vi "Calibration Main.vi"(8 "error in (no error)":errorcluster, 11 "Pump Calibration Config in":T1={"Settings"={"Cycle Period"=500.0, "Ismatech"={"VISA resource name"="", "Simulated?"=TRUE, "Pump Number"=1.0, "Reverse?"=FALSE}, "Masterflex"={"VISA resource name"="", "Simulated?"=TRUE, "Pump Number"=1.0, "Reverse?"=FALSE}, "Bronkhorst M13 Flow Meter"={"VISA resource name"="", "Simulated?"=TRUE}, "PID 2 Parameters"={"Input Device"=enum."Default", "Output Device"=enum."Default"}, "Bronkhorst M14"={"VISA resource name"="", "Simulated?"=FALSE}, "Tacmina Settings"={"Analog DAQ Task"="", "Digital DAQ Task"=""}, "KNF SIMDOS Settings"={"VISA resource name"="", "Simulated?"=TRUE}, "VICI M50 Settings"={"VISA resource name"="", "Simulated?"=TRUE, "Pump Letter"="", "Reverse?"=FALSE}, "FLOM Settings"={"VISA resource name"="", "Simulated?"=TRUE, "Pump Number"=0.0}, "Calibration Limits"={"Minimum (ml/min)"=0.0, "Maximum (ml/min)"=0.0, "Steps"=0.0}, "SSI PR Settings"={"VISA resource name"="", "Simulated?"=FALSE}}, "Flowmeter Output"=0.0, "Density"=0.0, "FL Temp"=0.0, "Speed %"=0.0, "File Refnum"=refnum, "Pump On?"=enum."Not Initialized"} {"Settings"."Masterflex"."Pump Number" min=1.0 max=20.0 step=1.0; "Settings"."Ismatech"."Pump Number" min=1.0 max=20.0 step=1.0}) -> (0 "error out":errorcluster, 3 "Pump Calibration Config out":T1={"Settings"={"Cycle Period"=500.0, "Ismatech"={"VISA resource name"="", "Simulated?"=TRUE, "Pump Number"=1.0, "Reverse?"=FALSE}, "Masterflex"={"VISA resource name"="", "Simulated?"=TRUE, "Pump Number"=1.0, "Reverse?"=FALSE}, "Bronkhorst M13 Flow Meter"={"VISA resource name"="", "Simulated?"=TRUE}, "PID 2 Parameters"={"Input Device"=enum."Default", "Output Device"=enum."Default"}, "Bronkhorst M14"={"VISA resource name"="", "Simulated?"=FALSE}, "Tacmina Settings"={"Analog DAQ Task"="", "Digital DAQ Task"=""}, "KNF SIMDOS Settings"={"VISA resource name"="", "Simulated?"=TRUE}, "VICI M50 Settings"={"VISA resource name"="", "Simulated?"=TRUE, "Pump Letter"="", "Reverse?"=FALSE}, "FLOM Settings"={"VISA resource name"="", "Simulated?"=TRUE, "Pump Number"=0.0}, "Calibration Limits"={"Minimum (ml/min)"=0.0, "Maximum (ml/min)"=0.0, "Steps"=0.0}, "SSI PR Settings"={"VISA resource name"="", "Simulated?"=FALSE}}, "Flowmeter Output"=0.0, "Density"=0.0, "FL Temp"=0.0, "Speed %"=0.0, "File Refnum"=refnum, "Pump On?"=enum."Not Initialized"} {"Settings"."Masterflex"."Pump Number" min=1.0 max=20.0 step=1.0; "Settings"."Ismatech"."Pump Number" min=1.0 max=20.0 step=1.0})   [LabVIEW 2018, in "Calibration.lvlib"]
uses:
  Pfizer Timed Seq/Software/Calibration VIs/Calibration.lvlib
  Pump Calibration Config.ctl
  Pfizer Timed Seq/Software/Ismatec ISM 831C/Controls/Ismatech Settings Cluster.ctl
  Pfizer Timed Seq/Software/Masterflex 7550-30/Controls/Settings Cluster.ctl
  Pfizer Timed Seq/Software/Bronkhorst M13 Flow Meter/Settings Cluster.ctl
  Pfizer Timed Seq/Software/Measure Instrument/PID Input Enum.ctl
  Pfizer Timed Seq/Software/Measure Instrument/PID 2 Output Enum.ctl
  Pfizer Timed Seq/Software/Mettler Toledo/Controls/Settings Cluster.ctl
  Pfizer Timed Seq/Software/Tacmina QI/Tacmina QI DAQ Setting.ctl
  Pfizer Timed Seq/Software/KNF Pump/Settings Cluster plus SIMDOS.ctl
  Pfizer Timed Seq/Software/VICI M50 Party Mode/Settings Cluster.ctl
  Pfizer Timed Seq/Software/FLOM Pump/Settings Cluster.ctl
  Pfizer Timed Seq/Software/SSI PR Class/SSI PR Settings Cluster.ctl
  Pfizer Timed Seq/Software/Bronkhorst M14 Flow Meter/Settings Cluster.ctl
  Pfizer Timed Seq/Software/ASIA Pump/Pump Settings.ctl
  <vilib>/Platform/TimedLoop/XDataNode/timing_clust.ctl
  <vilib>/Platform/TimedLoop/XDataNode/nitl_modes.ctl
  <vilib>/Platform/TimedLoop/XDataNode/wakeup.ctl
  Pfizer Timed Seq/Software/support/Message Queue/Enqueue Message (Single).vi
  <vilib>/Utility/file.llb/Read Delimited Spreadsheet (string).vi
  <vilib>/Utility/file.llb/Write Delimited Spreadsheet (string).vi
  <vilib>/Platform/TimedLoop/XDataNode/XDataNode.xnode
  <vilib>/regexp/Match Regular Expression.xnode
  Pfizer Timed Seq/Software/KNF Pump/KNF SIMDOS.lvlib
  Pfizer Timed Seq/Software/Ismatec ISM 831C/Ismatec ISM 831C.lvlib
  Pfizer Timed Seq/Software/VICI M50 Party Mode/VICI M6 M50 Party Mode.lvlib
  Pfizer Timed Seq/Software/Masterflex 7550-30/Masterflex 7550-30.lvlib
  Pfizer Timed Seq/Software/FLOM Pump/FLOM Pump.lvlib
  Pfizer Timed Seq/Software/Bronkhorst M13 Flow Meter/Bronkhorst M13 Flow Meter.lvlib
  Pfizer Timed Seq/Software/Bronkhorst M14 Flow Meter/Bronkhorst M14 Flow Meter.lvlib
  Pfizer Timed Seq/Software/support/Message Queue/Message Queue.lvlib
  Pfizer Timed Seq/Software/SSI PR Class/SSI PR Pump.lvlib
  Support/Engine.lvlib
  <vilib>/Analysis/NI_AALPro.lvlib
  <vilib>/Platform/TimedLoop/XDataNode/XDNodeRunTimeDep.lvlib
  Pfizer Timed Seq/Software/Mettler Toledo/Mettler Toledo.lvlib
  Pfizer Timed Seq/Software/Tacmina QI/Tacmina QI.lvlib
  Pfizer Timed Seq/Software/ASIA Pump.lvlib
panel:
  out "Y array":dbl[](array[numeric])
  out "X array":dbl[](array[numeric])
  out "Output Selected":bool
  out "Input Selected":bool
  out "Step Array":dbl[](array[numeric])
  in  "?":enum32{"Settings", "Results"}(tab)
  in  "Settings Dialog":T15={"Cycle Period"=500.0, "Ismatech"={"VISA resource name"="", "Simulated?"=FALSE, "Pump Number"=1.0, "Reverse?"=FALSE}, "Masterflex"={"VISA resource name"="", "Simulated?"=FALSE, "Pump Number"=1.0, "Reverse?"=FALSE}, "Mettler"={"VISA resource name"="", "Simulated?"=FALSE}, "Bronkhorst M13 Flow Meter"={"VISA resource name"="", "Simulated?"=FALSE}, "Setup Parameters"={"Input Device"=enum."Default", "Output Device"=enum."Default"}, "Bronkhorst M14 Settings"={"VISA resource name"="", "Simulated?"=FALSE}, "Tacmina Settings"={"Analog DAQ Task"="", "Digital DAQ Task"=""}, "KNF SIMDOS Settings"={"VISA resource name"="", "Simulated?"=FALSE}, "ASIA Pump C"={"ASIA Pump #"=-1, "channel"=-1, "Simulated"=FALSE}, "VICI M50 Settings"={"VISA resource name"="", "Simulated?"=FALSE, "Pump Letter"="", "Reverse?"=FALSE}, "FLOM Settings"={"VISA resource name"="", "Simulated?"=FALSE, "Pump Number"=1.0}, "Calibration Limits"={"Minimum (ml/min)"=0.0, "Maximum (ml/min)"=0.0, "Steps"=0.0}, "File Name"="", "SSI PR Settings"={"VISA resource name"="", "Simulated?"=FALSE}} {"Calibration Limits"."Maximum (ml/min)" max=16.5; "ASIA Pump C"."channel" min=-1 max=1 step=1; "Masterflex"."Pump Number" min=1.0 max=20.0 step=1.0; "Ismatech"."Pump Number" min=1.0 max=20.0 step=1.0}
  in  "Start Button":bool
  in  "Cancel Button":bool
  out "Y Intercept":dbl
  in  "Accept Button":bool
  in  "Decline Button":bool
  out "Calibration Graph":cluster{dbl[], dbl[]}[](graph)
  out "Calibration Slope":dbl
  out "R^2 Value":dbl format="%#.4g"
  out "Pump Status":enum16{"Off", "On", "Not Initialized"}(ring)
  # "Output Instruments"
  # "Input Instruments"
  # "Output Instruments"
  # "Input Instruments"
  # "Output Instruments"
  # "Input Instruments"
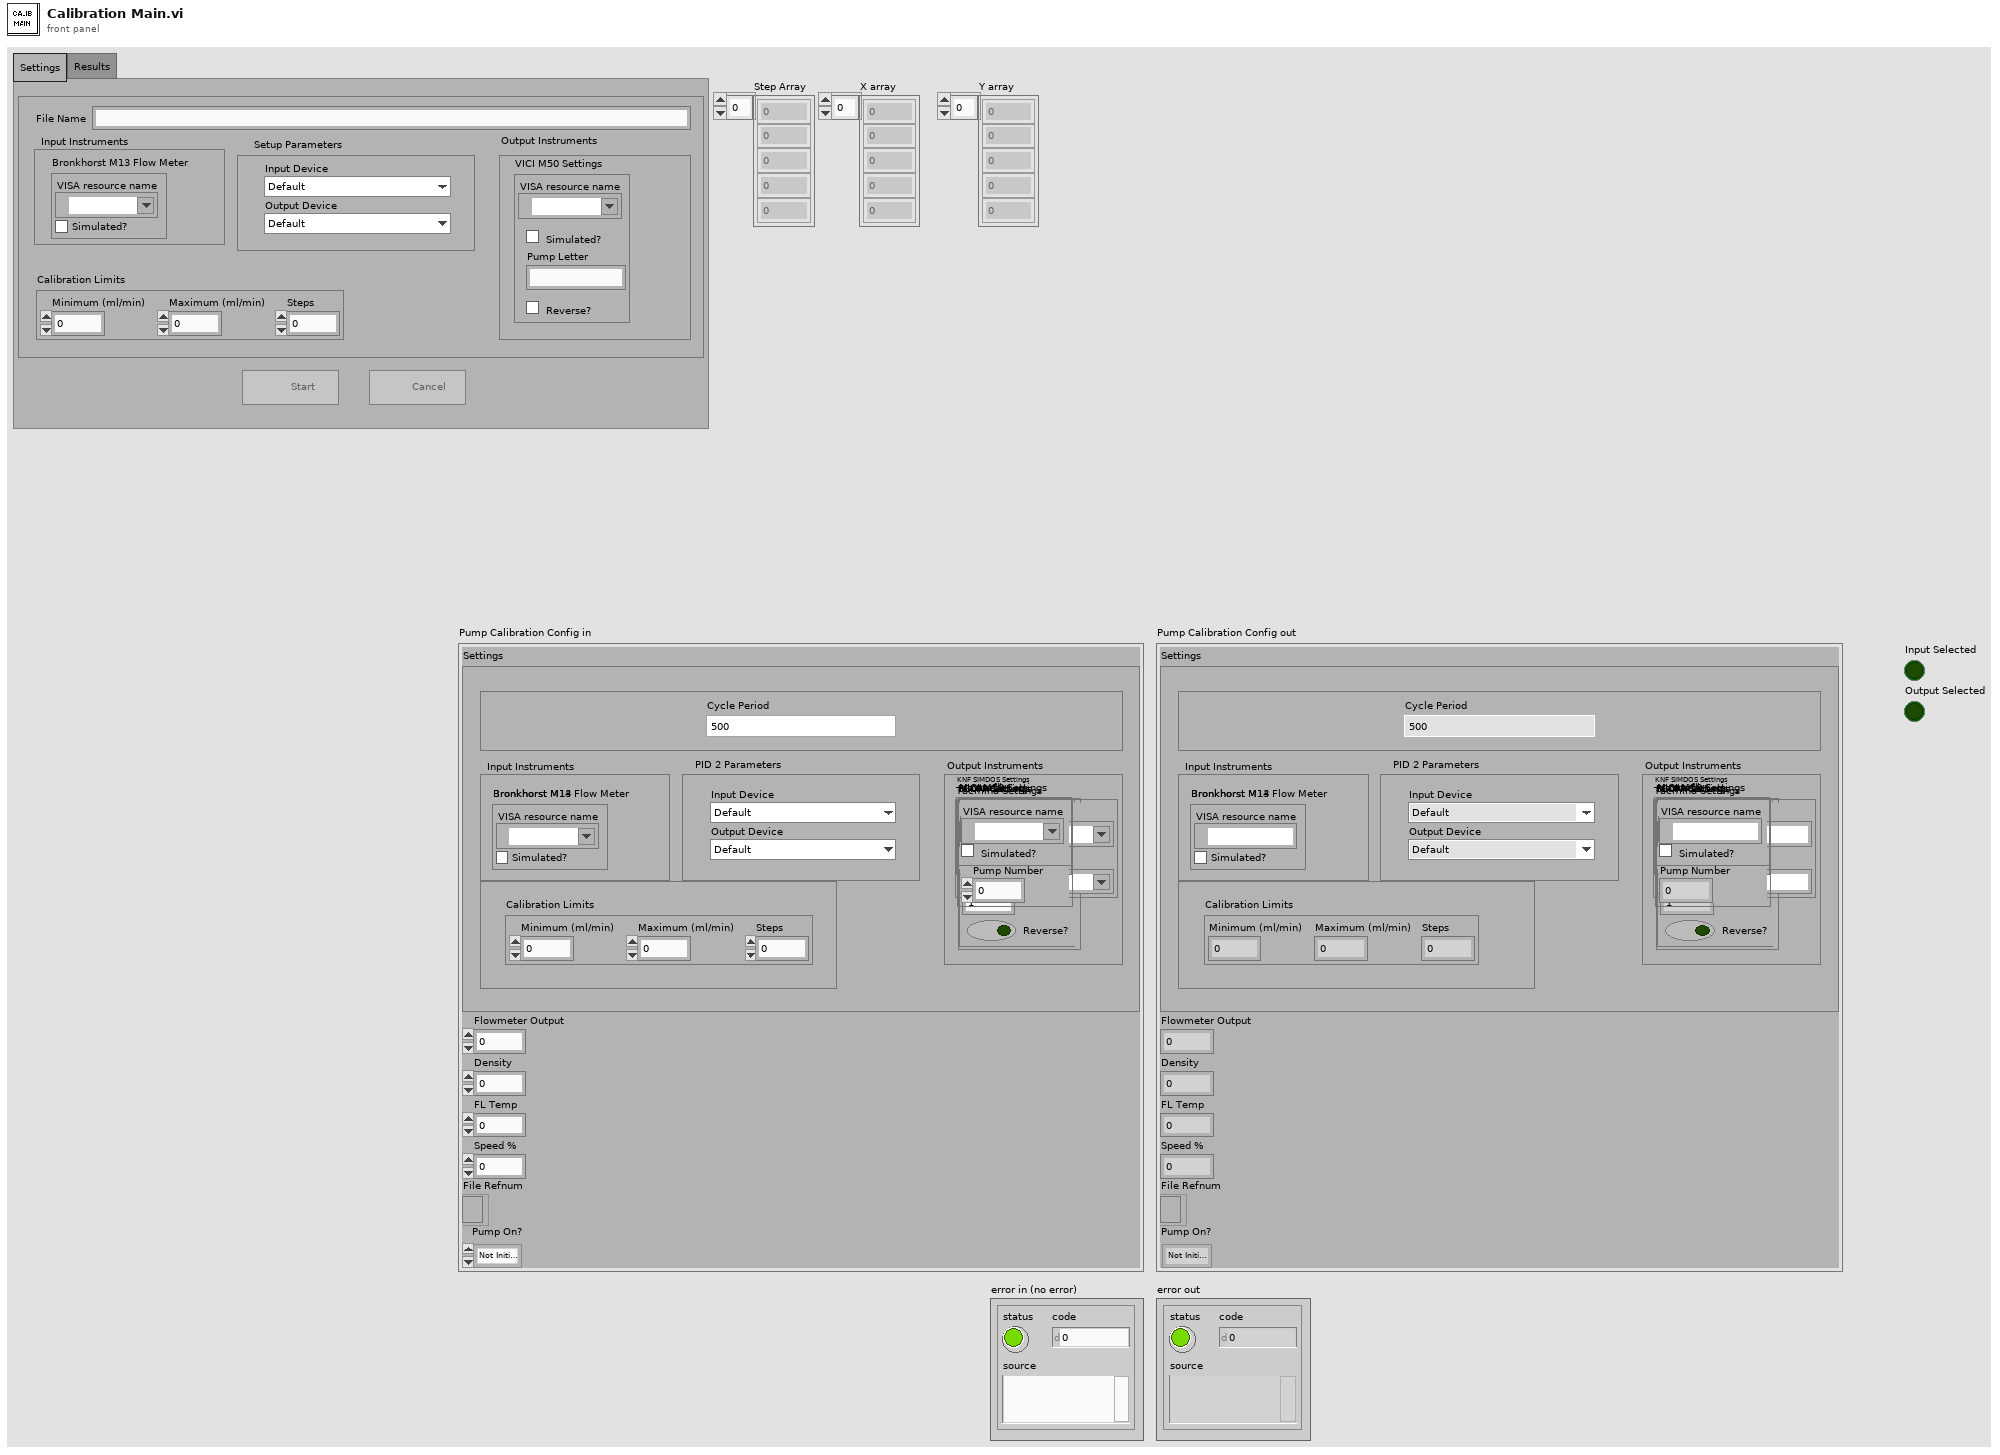
[diagram p1: front panel]
types:
  T1 = typedef "Calibration.lvlib/Pump Calibration Config.ctl" = cluster{"Settings":cluster{"Cycle Period":dbl, "Ismatech":T2, "Masterflex":T3, "Bronkhorst M13 Flow Meter":T4, "PID 2 Parameters":cluster{"Input Device":T5, "Output Device":T6}, "Bronkhorst M14":T7, "Tacmina Settings":T8, "KNF SIMDOS Settings":T9, "VICI M50 Settings":T10, "FLOM Settings":T11, "Calibration Limits":cluster{"Minimum (ml/min)":dbl, "Maximum (ml/min)":dbl, "Steps":dbl}, "SSI PR Settings":T12}, "Flowmeter Output":dbl, "Density":dbl, "FL Temp":dbl, "Speed %":dbl, "File Refnum":refnum<file>, "Pump On?":enum16{"Off", "On", "Not Initialized"}}
  T2 = typedef "Ismatec ISM 831C.lvlib/Ismatech Settings Cluster.ctl" = cluster{"VISA resource name":refnum<visa-resource-name>, "Simulated?":bool, "Pump Number":dbl, "Reverse?":bool}
  T3 = typedef "Masterflex 7550-30.lvlib/Settings Cluster.ctl" = cluster{"VISA resource name":refnum<visa-resource-name>, "Simulated?":bool, "Pump Number":dbl, "Reverse?":bool}
  T4 = typedef "Bronkhorst M13 Flow Meter.lvlib/Settings Cluster.ctl" = cluster{"VISA resource name":refnum<visa-resource-name>, "Simulated?":bool}
  T5 = typedef "PID Input Enum.ctl" = enum16{"Default", "Bronkhorst M13", "Bronkhorst M14", "Scale Rate of Change"}
  T6 = typedef "PID 2 Output Enum.ctl" = enum16{"Default", "Ismatec ISM 831C", "Masterflex 7550-30", "VICI", "Tacmina QI", "KNF SIMDOS", "ASIA Type C", "FLOM UI-22-11", "SSI PR"}
  T7 = typedef "Mettler Toledo.lvlib/Settings Cluster.ctl" = cluster{"VISA resource name":refnum<visa-resource-name>, "Simulated?":bool}
  T8 = typedef "Tacmina QI.lvlib/Tacmina QI DAQ Setting.ctl" = cluster{"Analog DAQ Task":refnum<k21>, "Digital DAQ Task":refnum<k21>}
  T9 = typedef "KNF SIMDOS.lvlib/Settings Cluster plus SIMDOS.ctl" = cluster{"VISA resource name":refnum<visa-resource-name>, "Simulated?":bool}
  T10 = typedef "VICI M6 M50 Party Mode.lvlib/Settings Cluster.ctl" = cluster{"VISA resource name":refnum<visa-resource-name>, "Simulated?":bool, "Pump Letter":string, "Reverse?":bool}
  T11 = typedef "FLOM Pump.lvlib/Settings Cluster.ctl" = cluster{"VISA resource name":refnum<visa-resource-name>, "Simulated?":bool, "Pump Number":dbl}
  T12 = typedef "SSI PR Pump.lvlib/SSI PR Settings Cluster.ctl" = cluster{"VISA resource name":refnum<visa-resource-name>, "Simulated?":bool}
  T13 = typedef "Bronkhorst M14 Flow Meter.lvlib/Settings Cluster.ctl" = cluster{"VISA resource name":refnum<visa-resource-name>, "Simulated?":bool}
  T14 = typedef "ASIA Pump.lvlib/Pump Settings.ctl" = cluster{"ASIA Pump #":i32, "channel":i32, "Simulated":bool}
  T15 = cluster{"Cycle Period":dbl, "Ismatech":T2, "Masterflex":T3, "Mettler":T7, "Bronkhorst M13 Flow Meter":T4, "Setup Parameters":cluster{"Input Device":T5, "Output Device":T6}, "Bronkhorst M14 Settings":T13, "Tacmina Settings":T8, "KNF SIMDOS Settings":T9, "ASIA Pump C":T14, "VICI M50 Settings":T10, "FLOM Settings":T11, "Calibration Limits":cluster{"Minimum (ml/min)":dbl, "Maximum (ml/min)":dbl, "Steps":dbl}, "File Name":string, "SSI PR Settings":T12}
  T16 = enum8{"Enabled", "Disabled", "Disabled and Grayed Out"}
  T17 = cluster{"Calibration UI":refnum<queue>, "Calibration Engine":refnum<queue>}
  T18 = typedef "XDNodeRunTimeDep.lvlib/timing_clust.ctl" = cluster{"Expected End [f-1]":u64, "Actual End [f-1]":u64, "Finished Late? [f-1]":bool, "Expected End [i-1]":u64, "Actual End [i-1]":u64, "Finished Late? [i-1]":bool, "Expected Start [i]":u64, "Actual Start [i]":u64, "Expected Start [f]":u64, "Actual Start [f]":u64, "Source Name":string, "Structure Name":string, "Period":i64, "Deadline":i64, "Offset":i64, "Start":i64, "Priority":i32, "Timeout":i32, "Mode":T19, "Wakeup Reason":T20, "Error":errorcluster, "Source Type":string, "Secondary Source Type":string, "Global End Time":u64, "Global Start Time":u64, "Frame Duration":u64, "Iteration Duration":u64, "Assigned CPU":i32, "I/O Scan Engine Mode":u32}
  T19 = typedef "XDNodeRunTimeDep.lvlib/nitl_modes.ctl" = enum32{"No Change", "Process missed periods, maintain original phase", "Discard missed periods, maintain original phase", "Process missed periods, ignore original phase", "Discard missed periods, ignore original phase"}
  T20 = typedef "XDNodeRunTimeDep.lvlib/wakeup.ctl" = enum32{"Normal", "Aborted", "Asynchronous wakeup", "Timing source error", "Timed loop error", "Timeout"}
  T21 = enum16{"open", "replace", "create", "open or create", "replace or create", "replace or create with confirmation"}
  T22 = cluster{"slope min":dbl, "slope max":dbl, "intercept min":dbl, "intercept max":dbl}
  T23 = cluster{"Minimum (ml/min)":dbl, "Maximum (ml/min)":dbl, "Steps":dbl}
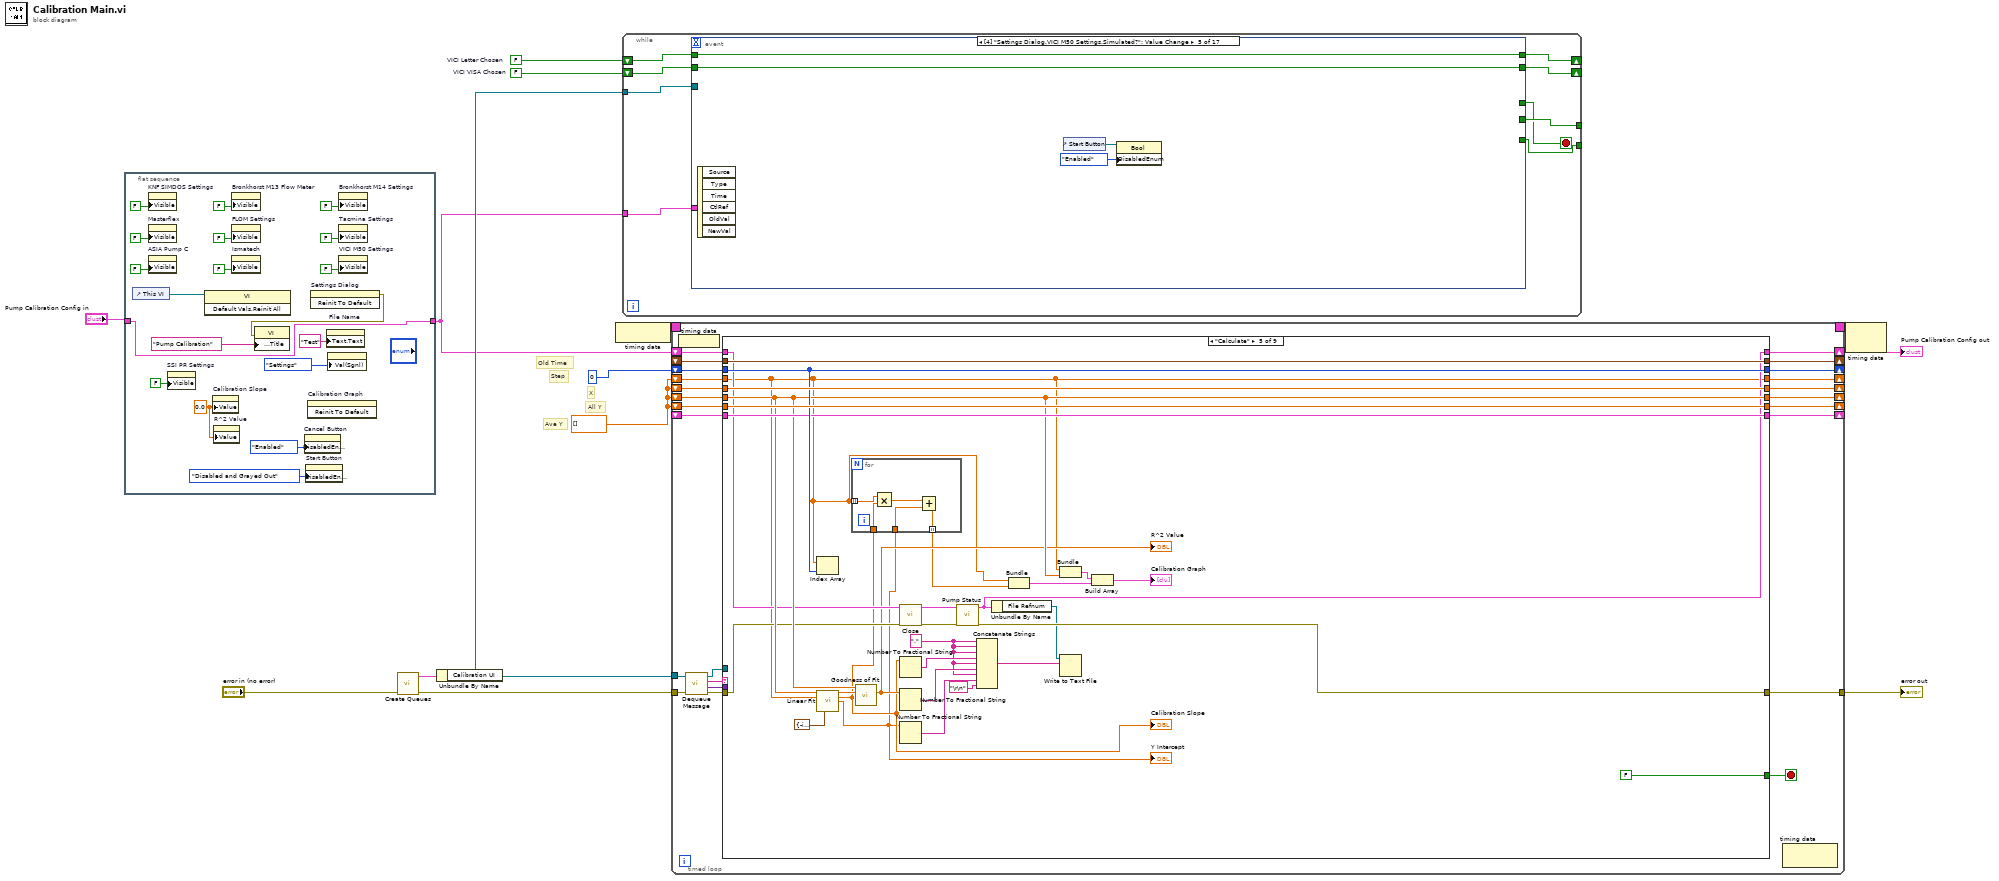
[diagram p0: block diagram]
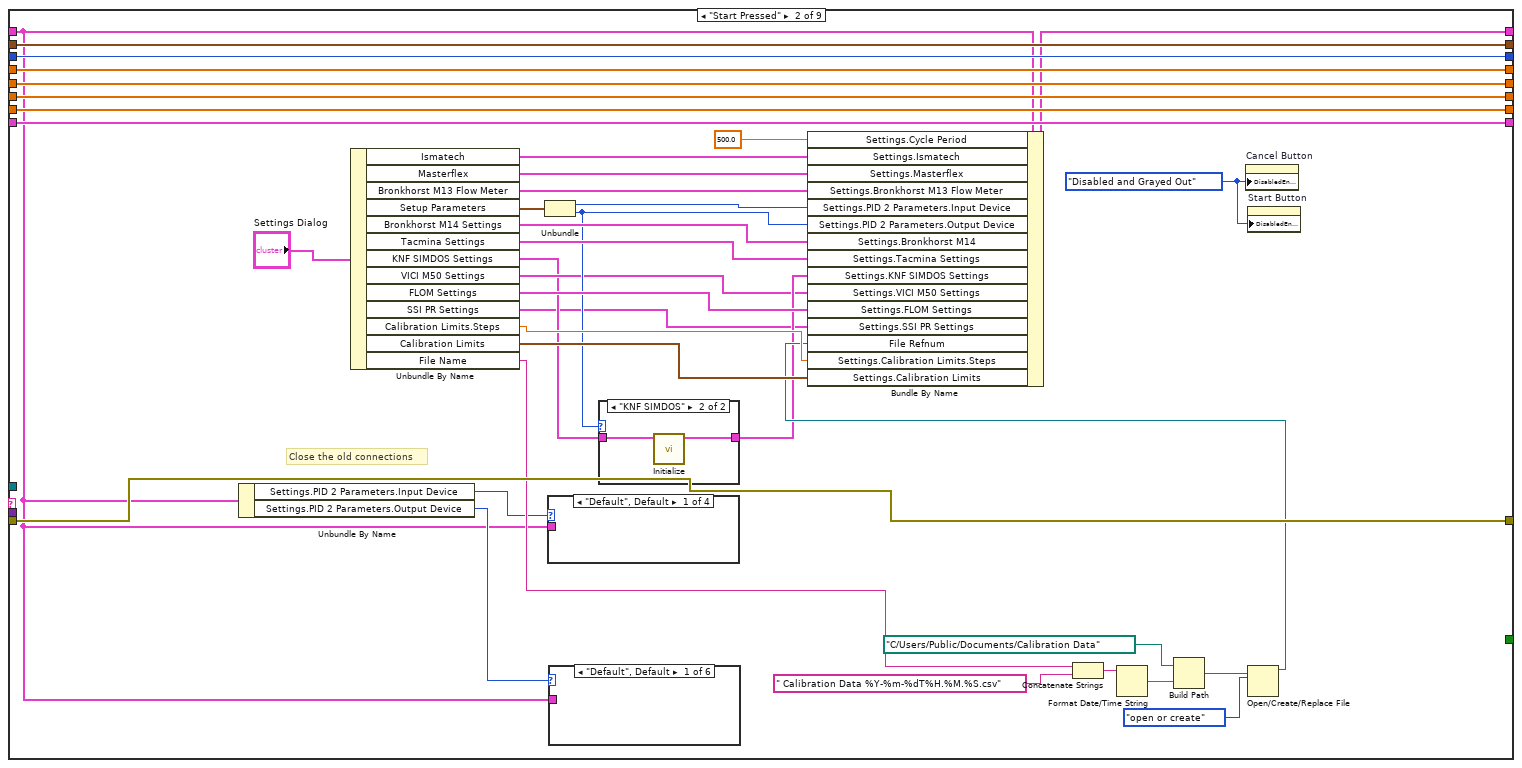
[diagram p3: hidden frame]
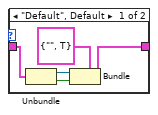
[diagram p4: hidden frame]
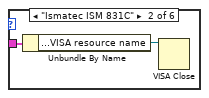
[diagram p5: hidden frame]
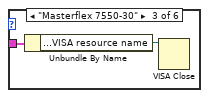
[diagram p6: hidden frame]
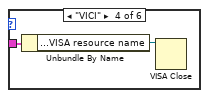
[diagram p7: hidden frame]
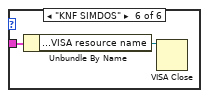
[diagram p9: hidden frame]
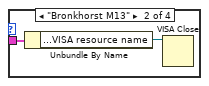
[diagram p10: hidden frame]
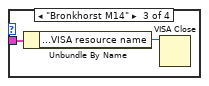
[diagram p11: hidden frame]
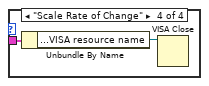
[diagram p12: hidden frame]
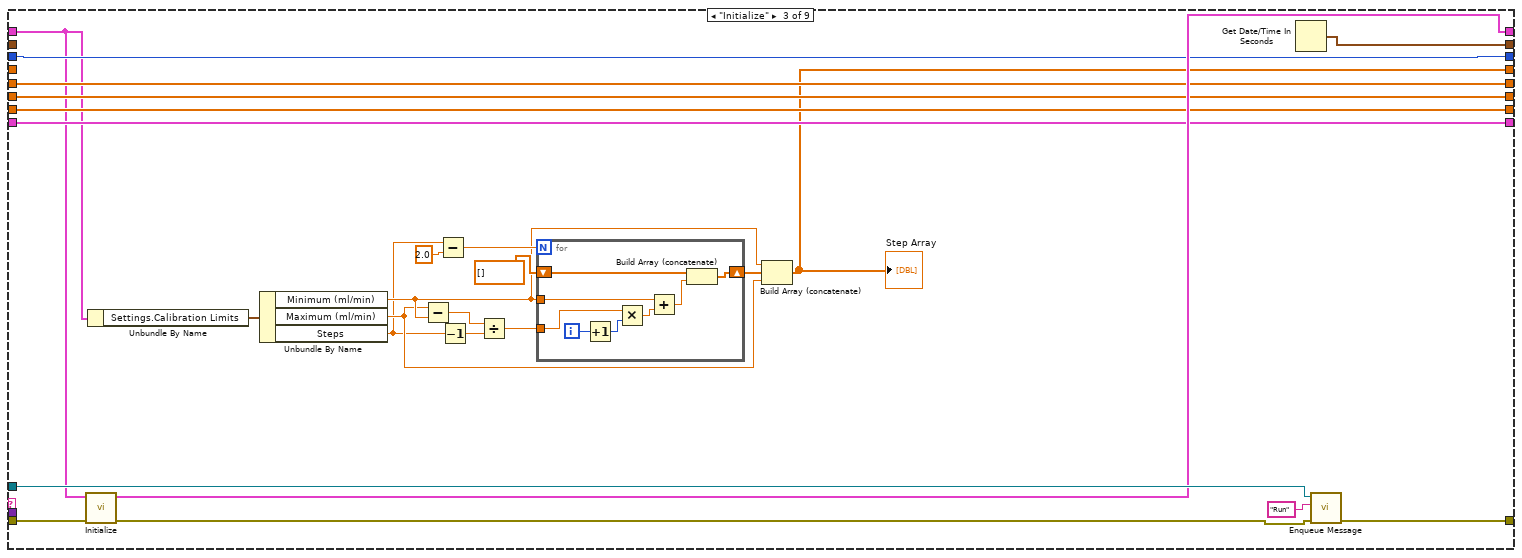
[diagram p13: hidden frame]
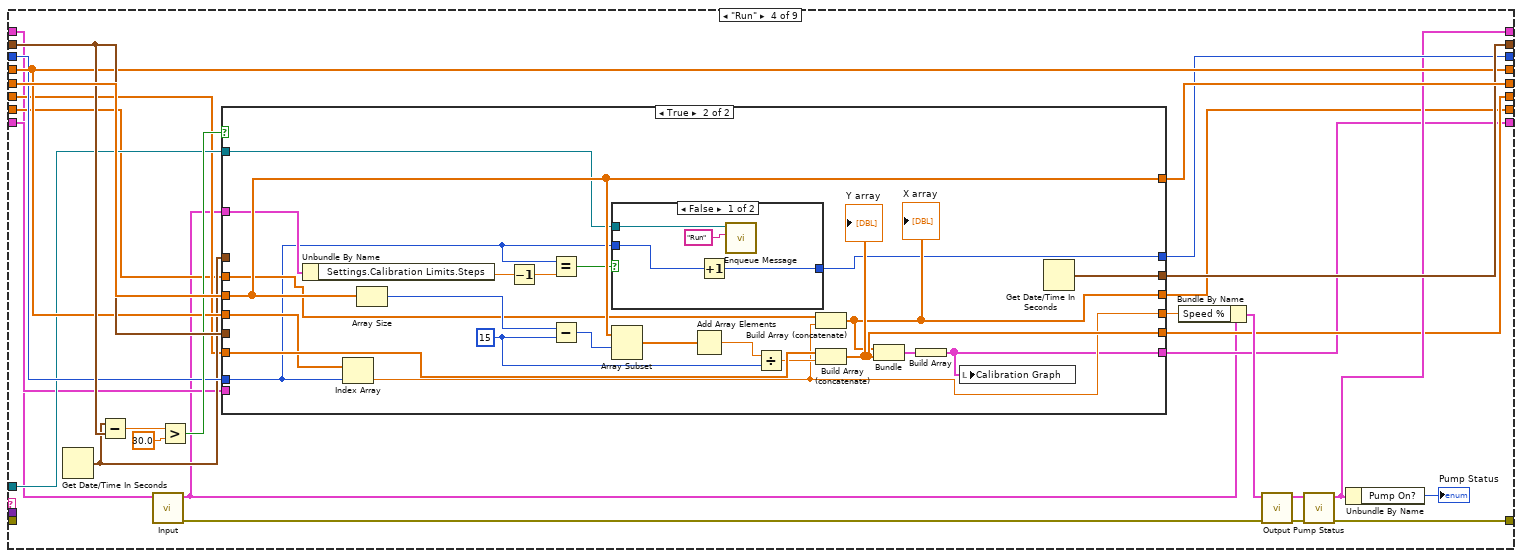
[diagram p14: hidden frame]
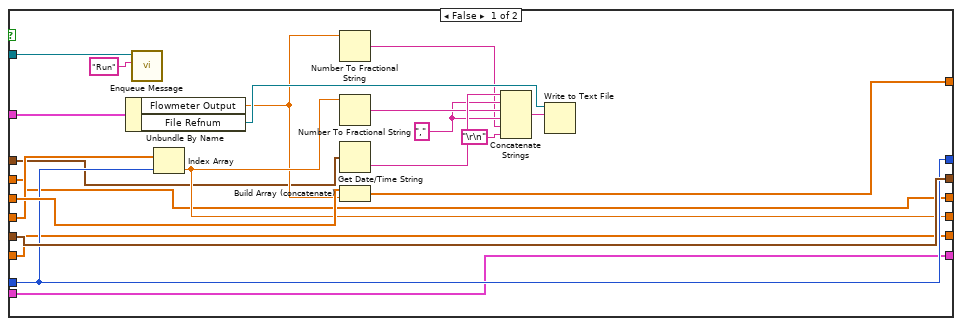
[diagram p15: hidden frame]
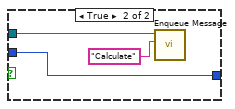
[diagram p16: hidden frame]
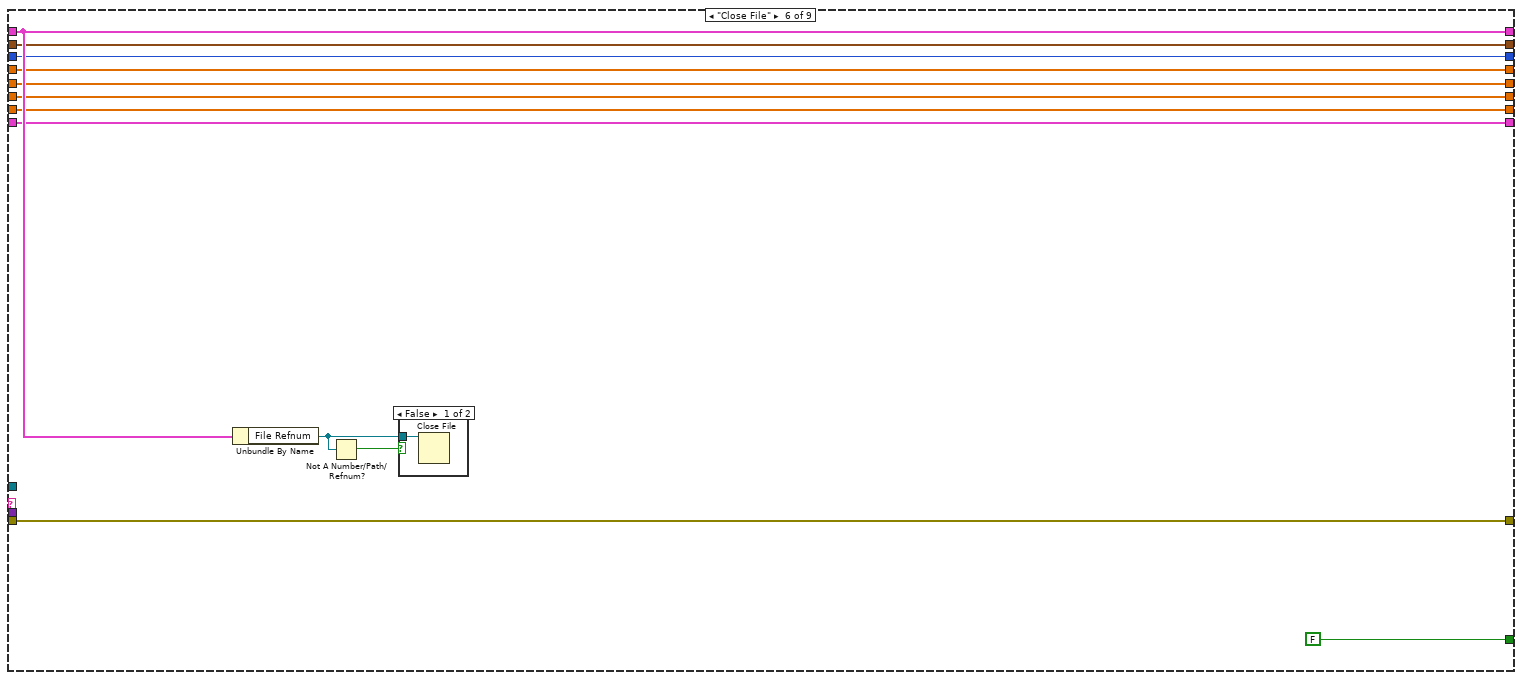
[diagram p17: hidden frame]
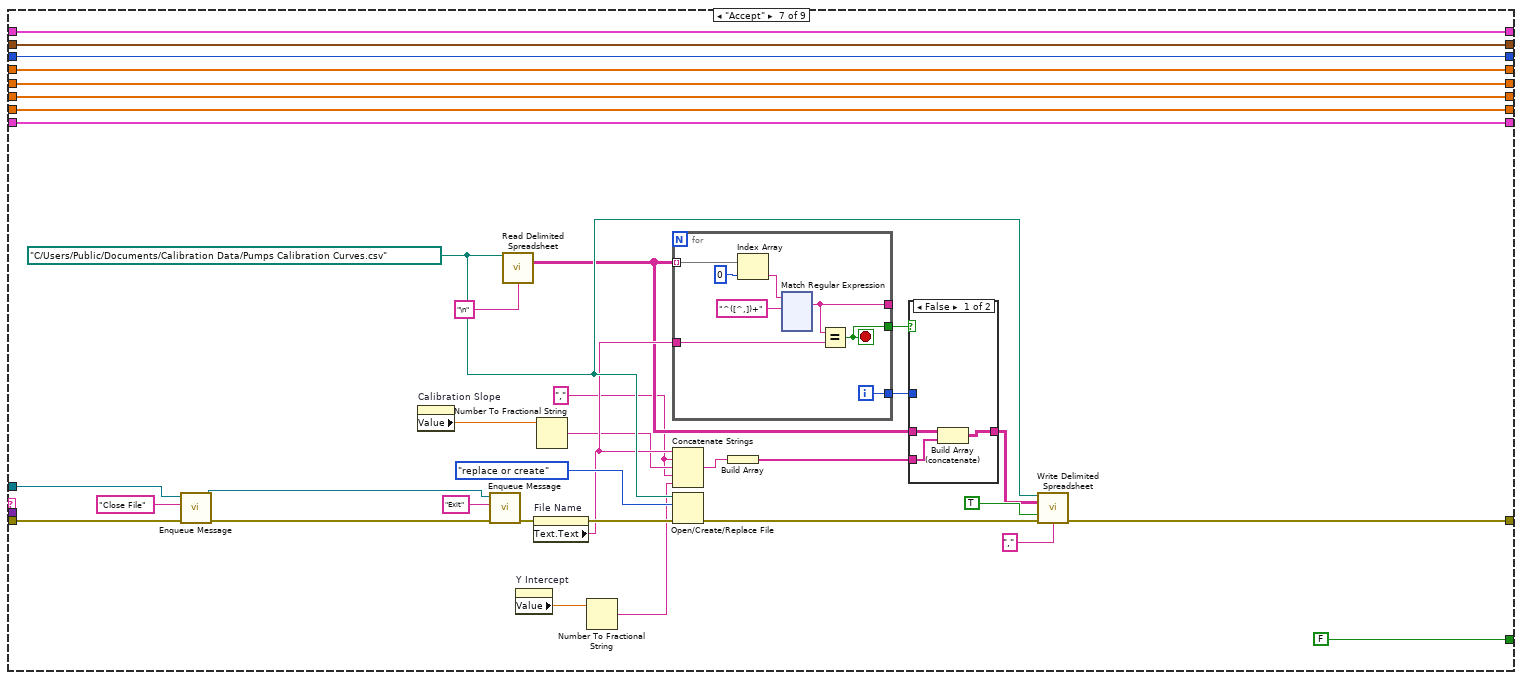
[diagram p19: hidden frame]
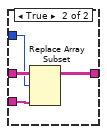
[diagram p20: hidden frame]
diagram:
  w1 = dbl[] []
  w13 = FALSE  # VICI VISA Chosen
  w14 = FALSE  # VICI Letter Chosen
  # "Old Time"
  # "Step"
  # "Ave Y"
  # "All Y"
  # "X"
  n1 = flat-sequence {
    tunnel: "Pump Calibration Config in" -> [w33]
    tunnel: [w33] -> w8
    frame #0 {
      w28 = 0.0 ("Calibration Slope")
      n2 = control-ref of="This VI"() -> (w27:refnum<vi>)
      n3 = property on="KNF SIMDOS Settings" class="Clust (strict)"("Visible"=FALSE) -> ()  [unwired: 2 in, 2 out]
      n4 = property on="Masterflex" class="Clust (strict)"("Visible"=FALSE) -> ()  [unwired: 2 in, 2 out]
      n5 = property on="ASIA Pump C" class="Clust (strict)"("Visible"=FALSE) -> ()  [unwired: 2 in, 2 out]
      n6 = property on="SSI PR Settings" class="Clust (strict)"("Visible"=FALSE) -> ()  [unwired: 2 in, 2 out]
      n7 = invoke class="VI" method="Default Vals.Reinit All"(reference=w27) -> ()  [unwired: 2 in, 3 out]
      n8 = property on="Calibration Slope" class="DigNum (strict)"("Value"=w28) -> ()  [unwired: 2 in, 2 out]
      n9 = property on="R^2 Value" class="DigNum (strict)"("Value"=w28) -> ()  [unwired: 2 in, 2 out]
      n10 = property on="Bronkhorst M13 Flow Meter" class="Clust (strict)"("Visible"=FALSE) -> ()  [unwired: 2 in, 2 out]
      n11 = property on="FLOM Settings" class="Clust (strict)"("Visible"=FALSE) -> ()  [unwired: 2 in, 2 out]
      n12 = property on="Ismatech" class="Clust (strict)"("Visible"=FALSE) -> ()  [unwired: 2 in, 2 out]
      n13 = property on="Cancel Button" class="Bool"("DisabledEnum"=T16."Enabled" ("Disabled")) -> ()  [unwired: 2 in, 2 out]
      n14 = property on="Start Button" class="Bool"("DisabledEnum"=T16."Disabled and Grayed Out" ("Disabled")) -> ()  [unwired: 2 in, 2 out]
      n15 = invoke on="Calibration Graph" class="XYGraph (strict)" method="Reinit To Default"() -> ()  [unwired: 3 in, 3 out]
      n16 = invoke on="Settings Dialog" class="Clust (strict)" method="Reinit To Default"() -> (error out=w30:errorcluster)  [unwired: 3 in, 2 out]
      n17 = property class="VI"(error in=w30, "Front Panel.Title"="Pump Calibration" ("string")) -> ()  [unwired: 1 in, 2 out]
      n18 = property on="File Name" class="Str"("Text.Text"="Test") -> ()  [unwired: 2 in, 2 out]
      n19 = property class="TabCtl (strict)"("Val(Sgnl)"=enum32{"Settings", "Results"}."Settings") -> ()  [unwired: 2 in, 2 out]
      n20 = property on="Bronkhorst M14 Settings" class="Clust (strict)"("Visible"=FALSE) -> ()  [unwired: 2 in, 2 out]
      n21 = property on="Tacmina Settings" class="Clust (strict)"("Visible"=FALSE) -> ()  [unwired: 2 in, 2 out]
      n22 = property on="VICI M50 Settings" class="Clust (strict)"("Visible"=FALSE) -> ()  [unwired: 2 in, 2 out]
    }
  }
  n23 = call "Create Queues.vi"("error in (no error)"="error in (no error)") -> ("error out"=w6:errorcluster, "Message Queues Out"=w10:T17)  [unwired: 9 in]
  n24 = Unbundle By Name(w10) -> ("Calibration UI"=w9:refnum<queue>)
  n25 = node-c288() -> (w4:T18)
  n26 = while {
    tunnel: [w42] -> _
    tunnel: [w40] -> _
    shift-right: [w39] -> _
    shift-left: w14 -> [w38]
    shift-right: [w37] -> _
    shift-left: w13 -> [w36]
    tunnel: w8 -> [w34]
    tunnel: w9 -> [w35]
    stop <- w41 stop-if-true
    n27 = event shown="[4] \"Settings Dialog.VICI M50 Settings.Simulated?\": Value Change" {
      selector: _ -> [_ _ _ _ _ _ _ _ _ _ _ _ _ _ _ _ _]
      dyn-events: _ -> [_ _ _ _ _ _ _ _ _ _ _ _ _ _ _ _ _]
      timeout: _ -> [_ _ _ _ _ _ _ _ _ _ _ _ _ _ _ _ _]
      tunnel: [FALSE ("UI Refresh Needed?") _ _ _ _ _ _ _ _ _ _ _ _ _ FALSE ("UI Refresh Needed?") FALSE ("UI Refresh Needed?") FALSE ("UI Refresh Needed?")] -> w42
      tunnel: [FALSE _ _ _ _ _ _ _ _ _ _ _ _ _ TRUE TRUE TRUE] -> w41
      tunnel: [FALSE ("UI Refresh Needed?") _ _ _ _ _ _ _ _ _ _ _ _ _ TRUE ("UI Refresh Needed?") TRUE ("UI Refresh Needed?") TRUE ("UI Refresh Needed?")] -> w40
      tunnel: [w49 w54 w66 TRUE w93 w98 w111 w128 w148 w163 w172 w186 w201 w220 w293 w300 w307] -> w39
      tunnel: w38 -> [w49 w54 w66 _ w93 w98 w111 w128 w148 w163 w172 w186 w201 w220 w293 w300 w307]
      tunnel: [w48 w53 TRUE w81 w96 w97 w110 w127 w147 w162 w171 w185 w200 w219 w292 w299 w306] -> w37
      tunnel: w36 -> [w48 w53 _ w81 w96 w97 w110 w127 w147 w162 w171 w185 w200 w219 w292 w299 w306]
      tunnel: w35 -> [w44 _ _ _ _ _ _ _ _ _ _ _ _ _ w290 w297 w304]
      tunnel: w34 -> [_ _ _ _ _ _ _ _ _ _ _ _ w199 w218 _ _ _]
      event "Start Button": Value Change {
        n28 = event-data() -> ()  [unwired: 1 in, 1 out]
        n29 = call-poly "Enqueue Message.vi"("Message"="Start Pressed", "Message Queue"=w44) -> ("dup Message Queue"=w43:refnum<queue>)  [unwired: 8 in, 1 out]
        n30 = property class="TabCtl (strict)"("Val(Sgnl)"=enum32{"Settings", "Results"}."Results") -> ()  [unwired: 2 in, 2 out]
        n31 = call-poly "Enqueue Message.vi"("Message"="Initialize", "Message Queue"=w43) -> ()  [unwired: 8 in, 2 out]
      }
      event Value Change {
        n32 = event-data() -> ("OldVal"=w56:refnum<visa-resource-name>)  [unwired: 1 in]
        n33 = local read "Settings Dialog"() -> (w59:T15)
        n34 = VISA Close(VISA resource name=w56) -> (error out=w57:errorcluster)  [unwired: 1 in]
        n35 = Unbundle By Name(w59) -> ("Ismatech"=w58:T2)
        n36 = call "Initialize.vi"("error in (no error)"=w57, "Ismatech Settings"=w58) -> ("No Pump Connected"=w55:bool)  [unwired: 6 in, 3 out]
        n37 = case shown="False" w55 {
          frame False {
            n38 = local read "Input Selected"() -> (w61:bool)
            n39 = case shown="True" w61 {
              frame False {
              }
              frame True {
                n40 = control-ref of="Start Button"() -> (w63:refnum<vi>)
                n41 = property on="Property Node" class="Bool"(reference=w63, "DisabledEnum"=T16."Enabled" ("Disabled")) -> ()  [unwired: 1 in, 2 out]
              }
            }
            "Output Selected" <- TRUE ("Output Selected")
          }
          frame True {
            n42 = control-ref of="Start Button"() -> (w64:refnum<vi>)
            n43 = property on="Property Node" class="Bool"(reference=w64, "DisabledEnum"=T16."Disabled and Grayed Out" ("Disabled")) -> ()  [unwired: 1 in, 2 out]
          }
        }
      }
      event Value Change {
        n44 = event-data() -> ("OldVal"=w68:refnum<visa-resource-name>)  [unwired: 1 in]
        n45 = local read "Settings Dialog"() -> (w71:T15)
        n46 = Unbundle By Name(w71) -> ("VICI M50 Settings"=w70:T10)
        n47 = VISA Close(VISA resource name=w68) -> (error out=w69:errorcluster)  [unwired: 1 in]
        n48 = case shown="True" w66 {
          tunnel: w70 -> [_ w74]
          tunnel: w69 -> [_ w73]
          frame False {
          }
          frame True {
            n49 = call "Initialize.vi"("error in (no error)"=w73, "VICI Settings"=w74) -> ("No Pump Connected"=w72:bool)  [unwired: 6 in, 3 out]
            n50 = case shown="False" w72 {
              frame False {
                n51 = local read "Input Selected"() -> (w75:bool)
                n52 = case shown="True" w75 {
                  frame False {
                  }
                  frame True {
                    n53 = control-ref of="Start Button"() -> (w78:refnum<vi>)
                    n54 = property on="Property Node" class="Bool"(reference=w78, "DisabledEnum"=T16."Enabled" ("Disabled")) -> ()  [unwired: 1 in, 2 out]
                  }
                }
                n55 = local write "Output Selected"(TRUE) -> ()
              }
              frame True {
                n56 = control-ref of="Start Button"() -> (w79:refnum<vi>)
                n57 = property on="Property Node" class="Bool"(reference=w79, "DisabledEnum"=T16."Disabled and Grayed Out" ("Disabled")) -> ()  [unwired: 1 in, 2 out]
              }
            }
          }
        }
      }
      event Value Change {
        n58 = event-data() -> ()  [unwired: 1 in, 1 out]
        n59 = local read "Settings Dialog"() -> (w84:T15)
        n60 = Unbundle By Name(w84) -> ("VICI M50 Settings"=w83:T10)
        n61 = case shown="True" w81 {
          tunnel: w83 -> [_ w86]
          frame False {
          }
          frame True {
            n62 = call "Initialize.vi"("VICI Settings"=w86) -> ("No Pump Connected"=w85:bool)  [unwired: 7 in, 3 out]
            n63 = case shown="False" w85 {
              frame False {
                n64 = local read "Input Selected"() -> (w87:bool)
                n65 = case shown="True" w87 {
                  frame False {
                  }
                  frame True {
                    n66 = control-ref of="Start Button"() -> (w90:refnum<vi>)
                    n67 = property on="Property Node" class="Bool"(reference=w90, "DisabledEnum"=T16."Enabled" ("Disabled")) -> ()  [unwired: 1 in, 2 out]
                  }
                }
                n68 = local write "Output Selected"(TRUE) -> ()
              }
              frame True {
                n69 = control-ref of="Start Button"() -> (w91:refnum<vi>)
                n70 = property on="Property Node" class="Bool"(reference=w91, "DisabledEnum"=T16."Disabled and Grayed Out" ("Disabled")) -> ()  [unwired: 1 in, 2 out]
              }
            }
          }
        }
      }
      event Value Change {
        n71 = event-data() -> ()  [unwired: 1 in, 6 out]
        n72 = control-ref of="Start Button"() -> (w95:refnum<vi>)
        n73 = property on="Property Node" class="Bool"(reference=w95, "DisabledEnum"=T16."Enabled" ("Disabled")) -> ()  [unwired: 1 in, 2 out]
      }
      event Value Change {
        n74 = event-data() -> ("OldVal"=w100:refnum<visa-resource-name>)  [unwired: 1 in]
        n75 = local read "Settings Dialog"() -> (w102:T15)
        n76 = VISA Close(VISA resource name=w100) -> (error out=w101:errorcluster)  [unwired: 1 in]
        n77 = Unbundle By Name(w102) -> ("Masterflex"=w103:T3)
        n78 = call "Initialize.vi"("error in (no error)"=w101, "Masterflex Settings in"=w103) -> ("No Pump Connected"=w99:bool)  [unwired: 6 in, 3 out]
        n79 = case shown="False" w99 {
          frame False {
            n80 = local read "Input Selected"() -> (w104:bool)
            n81 = case shown="True" w104 {
              frame False {
              }
              frame True {
                n82 = control-ref of="Start Button"() -> (w107:refnum<vi>)
                n83 = property on="Property Node" class="Bool"(reference=w107, "DisabledEnum"=T16."Enabled" ("Disabled")) -> ()  [unwired: 1 in, 2 out]
              }
            }
            n84 = local write "Output Selected"(TRUE) -> ()
          }
          frame True {
            n85 = control-ref of="Start Button"() -> (w108:refnum<vi>)
            n86 = property on="Property Node" class="Bool"(reference=w108, "DisabledEnum"=T16."Disabled and Grayed Out" ("Disabled")) -> ()  [unwired: 1 in, 2 out]
          }
        }
      }
      event Value Change {
        n87 = event-data() -> ("OldVal"=w115:refnum<visa-resource-name>)  [unwired: 1 in]
        n88 = local read "Settings Dialog"() -> (w116:T15)
        n89 = Unbundle By Name(w116) -> ("KNF SIMDOS Settings"=w113:T9)
        n90 = VISA Close(VISA resource name=w115) -> (error out=w114:errorcluster)  [unwired: 1 in]
        n91 = call "Initialize.vi"("error in (no error)"=w114, "KNF Settings"=w113) -> ("No Pump Connected"=w112:bool)  [unwired: 6 in, 3 out]
        n92 = case shown="False" w112 {
          frame False {
            n93 = local read "Input Selected"() -> (w117:bool)
            n94 = case shown="True" w117 {
              frame False {
              }
              frame True {
                n95 = control-ref of="Start Button"() -> (w120:refnum<vi>)
                n96 = property on="Property Node" class="Bool"(reference=w120, "DisabledEnum"=T16."Enabled" ("Disabled")) -> ()  [unwired: 1 in, 2 out]
              }
            }
            n97 = local write "Output Selected"(TRUE) -> ()
          }
          frame True {
            n98 = control-ref of="Start Button"() -> (w121:refnum<vi>)
            n99 = property on="Property Node" class="Bool"(reference=w121, "DisabledEnum"=T16."Disabled and Grayed Out" ("Disabled")) -> ()  [unwired: 1 in, 2 out]
          }
        }
      }
      event Value Change {
        n100 = event-data() -> ("OldVal"=w129:refnum<visa-resource-name>)  [unwired: 1 in]
        n101 = local read "Settings Dialog"() -> (w130:T15)
        n102 = Unbundle By Name(w130) -> ("FLOM Settings"=w124:T11)
        n103 = VISA Close(VISA resource name=w129) -> (error out=w126:errorcluster)  [unwired: 1 in]
        n104 = Unbundle By Name(w124) -> ("Pump Number"=w123:dbl)
        n105 = case shown="Default" w123 {
          tunnel: w126 -> [w134 _]
          tunnel: [w133 w137] -> _
          tunnel: [w132 FALSE ("Initialized")] -> w125
          tunnel: w124 -> [w131 w137]
          frame Default {
            n106 = call "Initialize.vi"("error in (no error)"=w134, "FLOM Settings in"=w131) -> ("Initialized"=w132:bool, "FLOM Settings out"=w133:T11)  [unwired: 6 in, 2 out]
          }
          frame 0 {
            n107 = One Button Dialog(message="Choose a Pump Number") -> ()  [unwired: 1 in, 1 out]
          }
        }
        n108 = case shown="True" w125 {
          frame False {
            n109 = control-ref of="Start Button"() -> (w138:refnum<vi>)
            n110 = property on="Property Node" class="Bool"(reference=w138, "DisabledEnum"=T16."Disabled and Grayed Out" ("Disabled")) -> ()  [unwired: 1 in, 2 out]
          }
          frame True {
            n111 = local read "Input Selected"() -> (w140:bool)
            n112 = case shown="True" w140 {
              frame False {
              }
              frame True {
                n113 = control-ref of="Start Button"() -> (w143:refnum<vi>)
                n114 = property on="Property Node" class="Bool"(reference=w143, "DisabledEnum"=T16."Enabled" ("Disabled")) -> ()  [unwired: 1 in, 2 out]
              }
            }
            n115 = local write "Output Selected"(TRUE) -> ()
          }
        }
      }
      event Value Change {
        n116 = event-data() -> ()  [unwired: 1 in, 1 out]
        n117 = local read "Settings Dialog"() -> (w149:T15)
        n118 = Unbundle By Name(w149) -> ("FLOM Settings"=w145:T11)
        n119 = Unbundle By Name(w145) -> ("Pump Number"=w144:dbl)
        n120 = case shown="Default" w144 {
          tunnel: [w151 FALSE ("Initialized")] -> w146
          tunnel: w145 -> [w150 _]
          frame Default {
            n121 = call "Initialize.vi"("FLOM Settings in"=w150) -> ("Initialized"=w151:bool)  [unwired: 7 in, 3 out]
          }
          frame 0 {
            n122 = One Button Dialog(message="Choose a non-zero Pump Number") -> ()  [unwired: 1 in, 1 out]
          }
        }
        n123 = case shown="True" w146 {
          frame False {
            n124 = control-ref of="Start Button"() -> (w154:refnum<vi>)
            n125 = property on="Property Node" class="Bool"(reference=w154, "DisabledEnum"=T16."Disabled and Grayed Out" ("Disabled")) -> ()  [unwired: 1 in, 2 out]
          }
          frame True {
            n126 = local read "Input Selected"() -> (w156:bool)
            n127 = case shown="True" w156 {
              frame False {
              }
              frame True {
                n128 = control-ref of="Start Button"() -> (w159:refnum<vi>)
                n129 = property on="Property Node" class="Bool"(reference=w159, "DisabledEnum"=T16."Enabled" ("Disabled")) -> ()  [unwired: 1 in, 2 out]
              }
            }
            n130 = local write "Output Selected"(TRUE) -> ()
          }
        }
      }
      event Value Change {
        n131 = event-data() -> ()  [unwired: 1 in, 1 out]
        n132 = local read "Settings Dialog"() -> (w164:T15)
        n133 = Unbundle By Name(w164) -> ("SSI PR Settings"=w160:T12)
        n134 = call "Initialize.vi"("SSI PR Settings In"=w160) -> ("Initialized"=w161:bool)  [unwired: 7 in, 3 out]
        n135 = case shown="True" w161 {
          frame False {
            n136 = control-ref of="Start Button"() -> (w165:refnum<vi>)
            n137 = property on="Property Node" class="Bool"(reference=w165, "DisabledEnum"=T16."Disabled and Grayed Out" ("Disabled")) -> ()  [unwired: 1 in, 2 out]
          }
          frame True {
            n138 = local read "Input Selected"() -> (w167:bool)
            n139 = case shown="True" w167 {
              frame False {
              }
              frame True {
                n140 = control-ref of="Start Button"() -> (w170:refnum<vi>)
                n141 = property on="Property Node" class="Bool"(reference=w170, "DisabledEnum"=T16."Enabled" ("Disabled")) -> ()  [unwired: 1 in, 2 out]
              }
            }
            n142 = local write "Output Selected"(TRUE) -> ()
          }
        }
      }
      event Value Change {
        n143 = event-data() -> ("OldVal"=w174:refnum<visa-resource-name>)  [unwired: 1 in]
        n144 = local read "Settings Dialog"() -> (w177:T15)
        n145 = Unbundle By Name(w177) -> ("Bronkhorst M13 Flow Meter"=w176:T4)
        n146 = VISA Close(VISA resource name=w174) -> (error out=w175:errorcluster)  [unwired: 1 in]
        n147 = call "Initialize.vi"("error in (no error)"=w175, "Bronkhorst Settings in"=w176) -> ("No Meter Connnected"=w173:bool)  [unwired: 7 in, 2 out]
        n148 = case shown="True" w173 {
          frame False {
            n149 = local read "Output Selected"() -> (w178:bool)
            n150 = case shown="True" w178 {
              frame False {
              }
              frame True {
                n151 = control-ref of="Start Button"() -> (w181:refnum<vi>)
                n152 = property on="Property Node" class="Bool"(reference=w181, "DisabledEnum"=T16."Enabled" ("Disabled")) -> ()  [unwired: 1 in, 2 out]
              }
            }
            "Input Selected" <- TRUE ("Input Selected")
          }
          frame True {
            n153 = control-ref of="Start Button"() -> (w183:refnum<vi>)
            n154 = property on="Property Node" class="Bool"(reference=w183, "DisabledEnum"=T16."Disabled and Grayed Out" ("Disabled")) -> ()  [unwired: 1 in, 2 out]
            n155 = local write "Input Selected"(FALSE ("Input Selected")) -> ()
          }
        }
      }
      event Value Change {
        n156 = event-data() -> ("OldVal"=w188:refnum<visa-resource-name>)  [unwired: 1 in]
        n157 = local read "Settings Dialog"() -> (w191:T15)
        n158 = Unbundle By Name(w191) -> ("Bronkhorst M14 Settings"=w190:T13)
        n159 = VISA Close(VISA resource name=w188) -> (error out=w189:errorcluster)  [unwired: 1 in]
        n160 = call "Initialize.vi"("error in (no error)"=w189, "Bronkhorst Settings in"=w190) -> ("No Meter Connected"=w187:bool)  [unwired: 7 in, 2 out]
        n161 = case shown="False" w187 {
          frame False {
            n162 = local read "Output Selected"() -> (w192:bool)
            n163 = case shown="True" w192 {
              frame False {
              }
              frame True {
                n164 = control-ref of="Start Button"() -> (w195:refnum<vi>)
                n165 = property on="Property Node" class="Bool"(reference=w195, "DisabledEnum"=T16."Enabled" ("Disabled")) -> ()  [unwired: 1 in, 2 out]
              }
            }
            n166 = local write "Input Selected"(TRUE ("Input Selected")) -> ()
          }
          frame True {
            n167 = property on="Start Button" class="Bool"("DisabledEnum"=T16."Disabled and Grayed Out" ("Disabled")) -> ()  [unwired: 2 in, 2 out]
            n168 = local write "Input Selected"(FALSE ("Input Selected")) -> ()
          }
        }
      }
      event Value Change {
        n169 = event-data() -> ("NewVal"=w202:T5)  [unwired: 1 in]
        n170 = case "Show the correct settings" shown="\"Bronkhorst M13\"" w202 {
          tunnel: w199 -> [w204 w210 _]
          tunnel: [16.5 ("Data Entry Limits:Maximum") 166.0 ("Data Entry Limits:Maximum") inf] -> w198
          frame "Bronkhorst M13" {
            n171 = Unbundle By Name(w204) -> ("Settings.Bronkhorst M13 Flow Meter.VISA resource name"=w206:refnum<visa-resource-name>)
            n172 = control-ref of="VISA resource name"() -> (w207:refnum<vi>)
            n173 = property on="Bronkhorst M14 Settings" class="Clust (strict)"("Visible"=FALSE) -> ()  [unwired: 2 in, 2 out]
            n174 = property on="Bronkhorst M13 Flow Meter" class="Clust (strict)"("Visible"=TRUE) -> ()  [unwired: 2 in, 2 out]
            n175 = property on="Property Node" class="VISAName"(reference=w207, "Value"=w206) -> ()  [unwired: 1 in, 2 out]
          }
          frame "Bronkhorst M14" {
            n176 = Unbundle By Name(w210) -> ("Settings.Bronkhorst M14.VISA resource name"=w212:refnum<visa-resource-name>)
            n177 = control-ref of="VISA resource name"() -> (w213:refnum<vi>)
            n178 = property on="Bronkhorst M14 Settings" class="Clust (strict)"("Visible"=TRUE) -> ()  [unwired: 2 in, 2 out]
            n179 = property on="Bronkhorst M13 Flow Meter" class="Clust (strict)"("Visible"=FALSE) -> ()  [unwired: 2 in, 2 out]
            n180 = property on="Property Node" class="VISAName"(reference=w213, "Value"=w212) -> ()  [unwired: 1 in, 2 out]
          }
          frame "Default", Default {
            n181 = property on="Bronkhorst M14 Settings" class="Clust (strict)"("Visible"=FALSE) -> ()  [unwired: 2 in, 2 out]
            n182 = property on="Bronkhorst M13 Flow Meter" class="Clust (strict)"("Visible"=FALSE) -> ()  [unwired: 2 in, 2 out]
          }
        }
        n183 = property on="Maximum (ml/min)" class="DigNum (strict)"("Maximum"=w198) -> ()  [unwired: 2 in, 2 out]
      }
      event Value Change {
        n184 = event-data() -> ("NewVal"=w221:T6)  [unwired: 1 in]
        n185 = case "Show the correct settings" shown="\"SSI PR\"" w221 {
          tunnel: w218 -> [w227 w237 w246 w257 _ _ _ w285]
          frame "Ismatec ISM 831C" {
            n186 = Unbundle By Name(w227) -> ("Settings.Ismatech.VISA resource name"=w228:refnum<visa-resource-name>)
            n187 = property on="VICI M50 Settings" class="Clust (strict)"("Visible"=FALSE) -> ()  [unwired: 2 in, 2 out]
            n188 = property on="Masterflex" class="Clust (strict)"("Visible"=FALSE) -> ()  [unwired: 2 in, 2 out]
            n189 = control-ref of="VISA resource name"() -> (w229:refnum<vi>)
            n190 = property on="Ismatech" class="Clust (strict)"("Visible"=TRUE) -> ()  [unwired: 2 in, 2 out]
            n191 = property on="FLOM Settings" class="Clust (strict)"("Visible"=FALSE) -> ()  [unwired: 2 in, 2 out]
            n192 = property on="Property Node" class="VISAName"(reference=w229, "Value"=w228) -> ()  [unwired: 1 in, 2 out]
            n193 = property on="KNF SIMDOS Settings" class="Clust (strict)"("Visible"=FALSE) -> ()  [unwired: 2 in, 2 out]
            n194 = property on="Tacmina Settings" class="Clust (strict)"("Visible"=FALSE) -> ()  [unwired: 2 in, 2 out]
            n195 = property on="SSI PR Settings" class="Clust (strict)"("Visible"=FALSE) -> ()  [unwired: 2 in, 2 out]
          }
          frame "FLOM UI-22-11" {
            n196 = Unbundle By Name(w237) -> ("Settings.FLOM Settings.VISA resource name"=w238:refnum<visa-resource-name>)
            n197 = property on="Ismatech" class="Clust (strict)"("Visible"=FALSE) -> ()  [unwired: 2 in, 2 out]
            n198 = property on="FLOM Settings" class="Clust (strict)"("Visible"=TRUE) -> ()  [unwired: 2 in, 2 out]
            n199 = property on="VICI M50 Settings" class="Clust (strict)"("Visible"=FALSE) -> ()  [unwired: 2 in, 2 out]
            n200 = property on="Masterflex" class="Clust (strict)"("Visible"=FALSE) -> ()  [unwired: 2 in, 2 out]
            n201 = control-ref of="VISA resource name"() -> (w239:refnum<vi>)
            n202 = property on="Property Node" class="VISAName"(reference=w239, "Value"=w238) -> ()  [unwired: 1 in, 2 out]
            n203 = property on="Tacmina Settings" class="Clust (strict)"("Visible"=FALSE) -> ()  [unwired: 2 in, 2 out]
            n204 = property on="KNF SIMDOS Settings" class="Clust (strict)"("Visible"=FALSE) -> ()  [unwired: 2 in, 2 out]
            n205 = property on="SSI PR Settings" class="Clust (strict)"("Visible"=FALSE) -> ()  [unwired: 2 in, 2 out]
          }
          frame "Masterflex 7550-30" {
            n206 = Unbundle By Name(w246) -> ("Settings.Masterflex.VISA resource name"=w247:refnum<visa-resource-name>)
            n207 = property on="Ismatech" class="Clust (strict)"("Visible"=FALSE) -> ()  [unwired: 2 in, 2 out]
            n208 = property on="FLOM Settings" class="Clust (strict)"("Visible"=FALSE) -> ()  [unwired: 2 in, 2 out]
            n209 = property on="VICI M50 Settings" class="Clust (strict)"("Visible"=FALSE) -> ()  [unwired: 2 in, 2 out]
            n210 = property on="Masterflex" class="Clust (strict)"("Visible"=TRUE) -> ()  [unwired: 2 in, 2 out]
            n211 = control-ref of="VISA resource name"() -> (w248:refnum<vi>)
            n212 = property on="Tacmina Settings" class="Clust (strict)"("Visible"=FALSE) -> ()  [unwired: 2 in, 2 out]
            n213 = property on="KNF SIMDOS Settings" class="Clust (strict)"("Visible"=FALSE) -> ()  [unwired: 2 in, 2 out]
            n214 = property on="Property Node" class="VISAName"(reference=w248, "Value"=w247) -> ()  [unwired: 1 in, 2 out]
          }
          frame "VICI" {
            n215 = property on="Ismatech" class="Clust (strict)"("Visible"=FALSE) -> ()  [unwired: 2 in, 2 out]
            n216 = property on="FLOM Settings" class="Clust (strict)"("Visible"=FALSE) -> ()  [unwired: 2 in, 2 out]
            n217 = Unbundle By Name(w257) -> ("Settings.VICI M50 Settings.VISA resource name"=w256:refnum<visa-resource-name>)
            n218 = property on="VICI M50 Settings" class="Clust (strict)"("Visible"=TRUE) -> ()  [unwired: 2 in, 2 out]
            n219 = property on="Masterflex" class="Clust (strict)"("Visible"=FALSE) -> ()  [unwired: 2 in, 2 out]
            n220 = property on="KNF SIMDOS Settings" class="Clust (strict)"("Visible"=FALSE) -> ()  [unwired: 2 in, 2 out]
            n221 = property on="Tacmina Settings" class="Clust (strict)"("Visible"=FALSE) -> ()  [unwired: 2 in, 2 out]
            n222 = property on="VISA resource name" class="VISAName"("Value"=w256) -> ()  [unwired: 2 in, 2 out]
            n223 = property on="SSI PR Settings" class="Clust (strict)"("Visible"=FALSE) -> ()  [unwired: 2 in, 2 out]
          }
          frame "Default", Default {
            n224 = property on="KNF SIMDOS Settings" class="Clust (strict)"("Visible"=FALSE) -> ()  [unwired: 2 in, 2 out]
            n225 = property on="FLOM Settings" class="Clust (strict)"("Visible"=FALSE) -> ()  [unwired: 2 in, 2 out]
            n226 = property on="Masterflex" class="Clust (strict)"("Visible"=FALSE) -> ()  [unwired: 2 in, 2 out]
            n227 = property on="Tacmina Settings" class="Clust (strict)"("Visible"=FALSE) -> ()  [unwired: 2 in, 2 out]
            n228 = property on="VICI M50 Settings" class="Clust (strict)"("Visible"=FALSE) -> ()  [unwired: 2 in, 2 out]
            n229 = property on="Ismatech" class="Clust (strict)"("Visible"=FALSE) -> ()  [unwired: 2 in, 2 out]
            n230 = property on="SSI PR Settings" class="Clust (strict)"("Visible"=FALSE) -> ()  [unwired: 2 in, 2 out]
          }
          frame "Tacmina QI" {
            n231 = property on="FLOM Settings" class="Clust (strict)"("Visible"=FALSE) -> ()  [unwired: 2 in, 2 out]
            n232 = property on="KNF SIMDOS Settings" class="Clust (strict)"("Visible"=FALSE) -> ()  [unwired: 2 in, 2 out]
            n233 = property on="Tacmina Settings" class="Clust (strict)"("Visible"=TRUE) -> ()  [unwired: 2 in, 2 out]
            n234 = property on="Ismatech" class="Clust (strict)"("Visible"=FALSE) -> ()  [unwired: 2 in, 2 out]
            n235 = property on="Masterflex" class="Clust (strict)"("Visible"=FALSE) -> ()  [unwired: 2 in, 2 out]
            n236 = property on="VICI M50 Settings" class="Clust (strict)"("Visible"=FALSE) -> ()  [unwired: 2 in, 2 out]
            n237 = property on="SSI PR Settings" class="Clust (strict)"("Visible"=FALSE) -> ()  [unwired: 2 in, 2 out]
          }
          frame "SSI PR" {
            n238 = property on="FLOM Settings" class="Clust (strict)"("Visible"=FALSE) -> ()  [unwired: 2 in, 2 out]
            n239 = property on="KNF SIMDOS Settings" class="Clust (strict)"("Visible"=FALSE) -> ()  [unwired: 2 in, 2 out]
            n240 = property on="Tacmina Settings" class="Clust (strict)"("Visible"=FALSE) -> ()  [unwired: 2 in, 2 out]
            n241 = property on="Ismatech" class="Clust (strict)"("Visible"=FALSE) -> ()  [unwired: 2 in, 2 out]
            n242 = property on="Masterflex" class="Clust (strict)"("Visible"=FALSE) -> ()  [unwired: 2 in, 2 out]
            n243 = property on="VICI M50 Settings" class="Clust (strict)"("Visible"=FALSE) -> ()  [unwired: 2 in, 2 out]
            n244 = property on="SSI PR Settings" class="Clust (strict)"("Visible"=TRUE) -> ()  [unwired: 2 in, 2 out]
          }
          frame "KNF SIMDOS" {
            n245 = property on="Ismatech" class="Clust (strict)"("Visible"=FALSE) -> ()  [unwired: 2 in, 2 out]
            n246 = property on="FLOM Settings" class="Clust (strict)"("Visible"=FALSE) -> ()  [unwired: 2 in, 2 out]
            n247 = Unbundle By Name(w285) -> ("Settings.KNF SIMDOS Settings.VISA resource name"=w286:refnum<visa-resource-name>)
            n248 = property on="VICI M50 Settings" class="Clust (strict)"("Visible"=FALSE) -> ()  [unwired: 2 in, 2 out]
            n249 = property on="Masterflex" class="Clust (strict)"("Visible"=FALSE) -> ()  [unwired: 2 in, 2 out]
            n250 = property on="Tacmina Settings" class="Clust (strict)"("Visible"=FALSE) -> ()  [unwired: 2 in, 2 out]
            n251 = property on="KNF SIMDOS Settings" class="Clust (strict)"("Visible"=TRUE) -> ()  [unwired: 2 in, 2 out]
            n252 = property on="VISA resource name" class="VISAName"("Value"=w286) -> ()  [unwired: 2 in, 2 out]
            n253 = property on="SSI PR Settings" class="Clust (strict)"("Visible"=FALSE) -> ()  [unwired: 2 in, 2 out]
          }
        }
      }
      event "Cancel Button": Value Change; Panel Close {
        # "True: Stop While Loop and Close Dialog"
        n254 = event-data() -> ()  [unwired: 1 in, 1 out]
        n255 = call-poly "Enqueue Message.vi"("Message"="Exit", "Message Queue"=w290) -> ()  [unwired: 8 in, 2 out]
      }
      event "Accept Button": Value Change {
        # "True: Stop While Loop and Close Dialog"
        n256 = event-data() -> ()  [unwired: 1 in, 1 out]
        n257 = call-poly "Enqueue Message.vi"("Message"="Accept", "Message Queue"=w297) -> ()  [unwired: 8 in, 2 out]
      }
      event "Decline Button": Value Change {
        # "True: Stop While Loop and Close Dialog"
        n258 = event-data() -> ()  [unwired: 1 in, 1 out]
        n259 = call-poly "Enqueue Message.vi"("Message"="Decline", "Message Queue"=w304) -> ()  [unwired: 8 in, 2 out]
      }
    }
  }
  n260 = timed-loop {
    tunnel: w9 -> [w334]
    shift-right: [w311] -> w5
    shift-left: w8 -> [w331]
    tunnel: [w330] -> w7
    tunnel: w6 -> [w327]
    shift-right: [w325] -> _
    shift-left: w1 -> [w324]
    timing: w4 -> [_]
    timing-out: [_] -> w3
    shift-right: [w323] -> _
    shift-left: w1 -> [w322]
    shift-right: [w321] -> _
    shift-left: _ -> [w320]
    shift-right: [w319] -> _
    shift-left: 0 -> [w318]
    shift-right: [w317] -> _
    shift-left: w1 -> [w316]
    shift-right: [w315] -> _
    shift-left: w1 -> [w314]
    shift-right: [w313] -> _
    shift-left: _ -> [w312]
    stop <- w329 stop-if-true
    n261 = node-c288() -> ()  [unwired: 1 in]
    n262 = call "Dequeue Message.vi"("error in (no error)"=w327, "Message Queue"=w334) -> ("error out"=w326:errorcluster, "Message Data"=w333:variant, "Message"=w332:string, "dup Message Queue"=w328:refnum<queue>)  [unwired: 6 in]
    n263 = case shown="\"Calculate\"" w332 {
      tunnel: w331 -> [w345 w354 w411 w440 w534 w561 w584 w744 w754]
      tunnel: w333 -> [_ _ _ _ _ _ _ _ _]
      tunnel: [w345 w353 w426 w448 w529 w561 w584 w744 w749] -> w311
      tunnel: [w344 w383 w414 w449 w530 w562 w582 w730 w755] -> w330
      tunnel: w326 -> [w344 w383 w427 _ w533 w562 w590 w734 w756]
      tunnel: [_ _ _ _ FALSE FALSE FALSE FALSE TRUE] -> w329
      tunnel: w328 -> [_ _ w428 w452 _ _ w591 w736 _]
      tunnel: [w343 w382 w408 w457 w517 w555 w596 w740 w753] -> w325
      tunnel: w324 -> [w343 w382 _ w457 w517 w555 w596 w740 w753]
      tunnel: [w342 w381 w420 w464 w545 w560 w599 w743 w752] -> w323
      tunnel: w322 -> [w342 w381 w420 w463 w545 w560 w599 w743 w752]
      tunnel: [w341 w380 w421 w460 w544 w559 w598 w742 w751] -> w321
      tunnel: w320 -> [w341 w380 _ w459 w544 w559 w598 w742 w751]
      tunnel: w318 -> [w340 w379 w419 w455 w538 w553 w594 w738 w750]
      tunnel: [w340 w379 w419 w453 w538 w553 w594 w738 w750] -> w319
      tunnel: [w339 w378 w418 w446 w536 w556 w597 w741 w748] -> w317
      tunnel: w316 -> [w339 w378 w418 w445 w536 w556 w597 w741 w748]
      tunnel: [w338 w377 w417 w444 w541 w554 w595 w739 w747] -> w315
      tunnel: w314 -> [w338 w377 w417 w443 w541 w554 w595 w739 w747]
      tunnel: [w337 w376 w416 w442 w537 w552 w593 w737 w746] -> w313
      tunnel: w312 -> [w337 w376 w416 w441 w537 w552 w593 w737 w746]
      frame Default {
      }
      frame "Start Pressed" {
        w352 = T16."Disabled and Grayed Out" ("Disabled")
        # "Close the old connections"
        n264 = Unbundle By Name(w354) -> ("Settings.PID 2 Parameters.Input Device"=w360:T5, "Settings.PID 2 Parameters.Output Device"=w361:T6)
        n265 = Unbundle By Name("Settings Dialog") -> ("Ismatech"=w355:T2, "Masterflex"=w356:T3, "Bronkhorst M13 Flow Meter"=w357:T4, "Setup Parameters"=w358:cluster{"Input Device":T5, "Output Device":T6}, "Bronkhorst M14 Settings"=w363:T13, "Tacmina Settings"=w364:T8, "KNF SIMDOS Settings"=w347:T9, "VICI M50 Settings"=w348:T10, "FLOM Settings"=w366:T11, "SSI PR Settings"=w346:T12, "Calibration Limits.Steps"=w373:dbl, "Calibration Limits"=w374:T23, "File Name"=w375:string)
        n266 = Unbundle(w358) -> ("Input Device"=w359:T5, "Output Device"=w362:T6)
        n267 = case shown="\"Default\", Default" w360 {
          tunnel: w354 -> [_ w400 w401 w403]
          frame "Default", Default {
          }
          frame "Bronkhorst M13" {
            n268 = Unbundle By Name(w400) -> ("Settings.Bronkhorst M13 Flow Meter.VISA resource name"=w399:refnum<visa-resource-name>)
            n269 = VISA Close(VISA resource name=w399) -> ()  [unwired: 1 in, 1 out]
          }
          frame "Bronkhorst M14" {
            n270 = Unbundle By Name(w401) -> ("Settings.Bronkhorst M14.VISA resource name"=w402:refnum<visa-resource-name>)
            n271 = VISA Close(VISA resource name=w402) -> ()  [unwired: 1 in, 1 out]
          }
          frame "Scale Rate of Change" {
            n272 = Unbundle By Name(w403) -> ("Settings.Ismatech.VISA resource name"=w404:refnum<visa-resource-name>)
            n273 = VISA Close(VISA resource name=w404) -> ()  [unwired: 1 in, 1 out]
          }
        }
        n274 = case shown="\"Default\", Default" w361 {
          tunnel: w354 -> [_ w391 w393 w395 _ w398]
          frame "Default", Default {
          }
          frame "Ismatec ISM 831C" {
            n275 = Unbundle By Name(w391) -> ("Settings.Ismatech.VISA resource name"=w392:refnum<visa-resource-name>)
            n276 = VISA Close(VISA resource name=w392) -> ()  [unwired: 1 in, 1 out]
          }
          frame "Masterflex 7550-30" {
            n277 = Unbundle By Name(w393) -> ("Settings.Masterflex.VISA resource name"=w394:refnum<visa-resource-name>)
            n278 = VISA Close(VISA resource name=w394) -> ()  [unwired: 1 in, 1 out]
          }
          frame "VICI" {
            n279 = Unbundle By Name(w395) -> ("Settings.Ismatech.VISA resource name"=w396:refnum<visa-resource-name>)
            n280 = VISA Close(VISA resource name=w396) -> ()  [unwired: 1 in, 1 out]
          }
          frame "Tacmina QI" {
            # "No VISA to Close"
          }
          frame "KNF SIMDOS" {
            n281 = Unbundle By Name(w398) -> ("Settings.KNF SIMDOS Settings.VISA resource name"=w397:refnum<visa-resource-name>)
            n282 = VISA Close(VISA resource name=w397) -> ()  [unwired: 1 in, 1 out]
          }
        }
        n283 = case shown="\"KNF SIMDOS\"" w362 {
          tunnel: w347 -> [w388 w389]
          tunnel: [w387 w390] -> w365
          frame "Default", Default {
            n284 = Unbundle(w388) -> ("VISA resource name"=w385:refnum<visa-resource-name>, "Simulated?"=w384:bool)
            n285 = Bundle(cluster=T9 {"VISA resource name"="", "Simulated?"=TRUE} ("KNF Settings"), "VISA resource name"=w385, "Simulated?"=w384) -> (w387:T9)
          }
          frame "KNF SIMDOS" {
            n286 = call "Initialize.vi"("KNF Settings"=w389) -> ("KNF Settings"=w390:T9)  [unwired: 7 in, 3 out]
          }
        }
        n287 = Concatenate Strings(w375, " Calibration Data %Y-%m-%dT%H.%M.%S.csv" ("time format string (%c)")) -> (w370:string)
        n288 = Format Date/Time String(time format string (%c)=w370) -> (date/time string=w351:string)  [unwired: 2 in]
        n289 = Build Path(base path=path "C:/Users/Public/Documents/Calibration Data", name or relative path=w351) -> (appended path=w350:path)
        n290 = property on="Cancel Button" class="Bool"("DisabledEnum"=w352) -> ()  [unwired: 2 in, 2 out]
        n291 = property on="Start Button" class="Bool"("DisabledEnum"=w352) -> ()  [unwired: 2 in, 2 out]
        n292 = Open/Create/Replace File(file path (use dialog)=w350, operation (0:open)=T21."open or create") -> (refnum out=w372:refnum<file>)  [unwired: 4 in, 2 out]
        n293 = Bundle By Name(cluster=w354, "Settings.Cycle Period"=500.0, "Settings.Ismatech"=w355, "Settings.Masterflex"=w356, "Settings.Bronkhorst M13 Flow Meter"=w357, "Settings.PID 2 Parameters.Input Device"=w359, "Settings.PID 2 Parameters.Output Device"=w362, "Settings.Bronkhorst M14"=w363, "Settings.Tacmina Settings"=w364, "Settings.KNF SIMDOS Settings"=w365, "Settings.VICI M50 Settings"=w348, "Settings.FLOM Settings"=w366, "Settings.SSI PR Settings"=w346, "File Refnum"=w372, "Settings.Calibration Limits.Steps"=w373, "Settings.Calibration Limits"=w374) -> (w353:T1)
      }
      frame "Initialize" {
        n294 = call "Initialize.vi"("error in"=w427, "Pump Calibration Config in"=w411) -> ("error out"=w415:errorcluster, "Pump Calibration Config Out"=w426:T1)  [unwired: 8 in]
        n295 = Unbundle By Name(w411) -> ("Settings.Calibration Limits"=w425:T23)
        n296 = Unbundle By Name(w425) -> ("Minimum (ml/min)"=w409:dbl, "Maximum (ml/min)"=w407:dbl, "Steps"=w406:dbl)
        n297 = Subtract(x=w407, y=w409) -> (x-y=w424:dbl)
        n298 = Subtract(x=w406, y=2.0) -> (x-y=w412:dbl)
        n299 = Decrement(x=w406) -> (x-1=w405:dbl)
        n300 = Divide(x=w424, y=w405) -> (x/y=w422:dbl)
        n301 = for {
          N: w412 -> [_]
          shift-right: [w434] -> w410
          shift-left: dbl[] [] -> [w435]
          tunnel: w409 -> [w433]
          tunnel: w422 -> [w432]
          i -> [w431]
          n302 = Increment(x=w431) -> (x+1=w430:i32)
          n303 = Multiply(x=w432, y=w430) -> (x*y=w437:dbl)
          n304 = Add(x=w433, y=w437) -> (x+y=w436:dbl)
          n305 = Build Array (concatenate)(w435, w436) -> (w434:dbl[])
        }
        n306 = Build Array (concatenate)(w409, w410, w407) -> (w408:dbl[])
        "Step Array" <- w408
        n307 = Get Date/Time In Seconds() -> (seconds since 1Jan1904=w421:timestamp)
        n308 = call-poly "Enqueue Message.vi"("error in (no error)"=w415, "Message"="Run", "Message Queue"=w428) -> ("error out"=w414:errorcluster)  [unwired: 7 in, 1 out]
      }
      frame "Run" {
        n309 = Get Date/Time In Seconds() -> (seconds since 1Jan1904=w451:timestamp)
        n310 = Subtract(x=w451, y=w459) -> (x-y=w462:dbl)
        n311 = call "Input.vi"("Pump Calibration Config in"=w440) -> ("error out"=w465:errorcluster, "Pump Calibration Config Out"=w439:T1)  [unwired: 9 in]
        n312 = Greater?(x=w462, y=30.0) -> (0:w458:bool)
        n313 = case shown="True" w458 {
          tunnel: w439 -> [w484 w501]
          tunnel: [w485 w506] -> w464
          tunnel: w463 -> [w486 w506]
          tunnel: [w483 w509] -> w460
          tunnel: w459 -> [w483 _]
          tunnel: w457 -> [w482 w497]
          tunnel: w455 -> [w481 w492]
          tunnel: [w477 w495] -> w454
          tunnel: [w481 w491] -> w453
          tunnel: w452 -> [w480 w502]
          tunnel: w451 -> [w475 _]
          tunnel: [w468 w496] -> w446
          tunnel: w445 -> [w468 w499]
          tunnel: [w467 w493] -> w444
          tunnel: w443 -> [w467 w494]
          tunnel: [w466 w489] -> w442
          tunnel: w441 -> [w466 _]
          frame False {
            w471 = "," ("string")
            n314 = Unbundle By Name(w484) -> ("Flowmeter Output"=w476:dbl, "File Refnum"=w479:refnum<file>)
            n315 = call-poly "Enqueue Message.vi"("Message"="Run", "Message Queue"=w480) -> ()  [unwired: 8 in, 2 out]
            n316 = Index Array(array=w482, index=w481) -> (element=w477:dbl)
            n317 = Number To Fractional String(number=w476) -> (F-format string=w470:string)  [unwired: 3 in]
            n318 = Number To Fractional String(number=w477) -> (F-format string=w472:string)  [unwired: 3 in]
            n319 = Get Date/Time String(seconds (now)=w475) -> (time string=w473:string)  [unwired: 2 in, 1 out]
            n320 = Build Array (concatenate)(w486, w476) -> (w485:dbl[])
            n321 = Concatenate Strings(w473, w471, w472, w471, w470, "\r\n") -> (w478:string)
            n322 = Write to Text File(file (use dialog)=w479, text=w478) -> ()  [unwired: 2 in, 3 out]
          }
          frame True {
            w503 = 15 ("y")
            n323 = Unbundle By Name(w501) -> ("Settings.Calibration Limits.Steps"=w487:dbl)
            n324 = Index Array(array=w497, index=w492) -> (element=w495:dbl)
            n325 = Array Size(array=w506) -> (size(s)=w508:i32)
            n326 = Decrement(x=w487) -> (x-1=w488:dbl)
            n327 = Equal?(x=w492, y=w488) -> (x = y?=w500:bool)
            n328 = Subtract(x=w508, y=w503) -> (x-y=w507:i32)
            n329 = case shown="False" w500 {
              tunnel: w502 -> [w512 w516]
              tunnel: w492 -> [w511 w515]
              tunnel: [w510 w515] -> w491
              frame False {
                n330 = Increment(x=w511) -> (x+1=w510:i32)
                n331 = call-poly "Enqueue Message.vi"("Message"="Run", "Message Queue"=w512) -> ()  [unwired: 8 in, 2 out]
              }
              frame True {
                n332 = call-poly "Enqueue Message.vi"("Message"="Calculate", "Message Queue"=w516) -> ()  [unwired: 8 in, 2 out]
              }
            }
            n333 = Array Subset(array=w506, index=w507) -> (w505:dbl[])  [unwired: 1 in]
            n334 = Add Array Elements(numeric array=w505) -> (sum=w504:dbl)
            n335 = Divide(x=w504, y=w503) -> (x/y=w498:dbl)
            n336 = Build Array (concatenate)(w494, w495) -> (w493:dbl[])
            "X array" <- w493
            n337 = Build Array (concatenate)(w499, w498) -> (w496:dbl[])
            "Y array" <- w496
            n338 = Bundle(w493, w496) -> (w490:cluster{dbl[], dbl[]})  [unwired: 1 in]
            n339 = Build Array(w490) -> (w489:cluster{dbl[], dbl[]}[])
            n340 = local write "Calibration Graph"(w489) -> ()
            n341 = Get Date/Time In Seconds() -> (seconds since 1Jan1904=w509:timestamp)
          }
        }
        n342 = Bundle By Name(cluster=w439, "Speed %"=w454) -> (w456:T1)
        n343 = call "Output.vi"("error in (no error)"=w465, "Pump Calibration Config in"=w456) -> ("error out"=w450:errorcluster, "Pump Calibration Config Out"=w438:T1)  [unwired: 8 in]
        n344 = call "Pump Status.vi"("error in (no error)"=w450, "Pump Calibration Config in"=w438) -> ("error out"=w449:errorcluster, "Pump Calibration Config out"=w448:T1)  [unwired: 8 in]
        n345 = Unbundle By Name(w448) -> ("Pump On?"=→"Pump Status":enum16{"Off", "On", "Not Initialized"})
      }
      frame "Calculate" {
        w522 = "," ("string")
        n346 = Index Array(array=w517, index=w538) -> ()  [unwired: 1 out]
        n347 = call <vilib>:"Linear Fit.vi"("Y"=w536, "X"=w517, "parameter bounds"=T22 {"slope min"=-inf, "slope max"=inf, "intercept min"=-inf, "intercept max"=inf}) -> ("Best Linear Fit"=w535:dbl[], "slope"=w520:dbl, "intercept"=w519:dbl)  [unwired: 8 in, 2 out]
        "Calibration Slope" <- w520
        "Y Intercept" <- w519
        n348 = for {
          tunnel: w517 -> [w550] mode=indexing
          tunnel: w520 -> [w549]
          tunnel: w519 -> [w548]
          tunnel: [w547] -> w518 mode=indexing
          n349 = Multiply(x=w550, y=w549) -> (x*y=w551:dbl)
          n350 = Add(x=w551, y=w548) -> (x+y=w547:dbl)
        }
        n351 = call <vilib>:"Goodness of Fit.vi"("Best Fit"=w535, "Y"=w536) -> ("R-square"=w525:dbl)  [unwired: 6 in, 3 out]
        "R^2 Value" <- w525
        n352 = call "Close.vi"("error in (no error)"=w533, "Pump Calibration Config in"=w534) -> ("error out"=w531:errorcluster, "Pump Calibration Config out"=w532:T1)  [unwired: 8 in]
        n353 = Number To Fractional String(number=w520) -> (F-format string=w526:string)  [unwired: 3 in]
        n354 = Number To Fractional String(number=w525) -> (F-format string=w524:string)  [unwired: 3 in]
        n355 = Number To Fractional String(number=w519) -> (F-format string=w521:string)  [unwired: 3 in]
        n356 = call "Pump Status.vi"("error in (no error)"=w531, "Pump Calibration Config in"=w532) -> ("error out"=w530:errorcluster, "Pump Calibration Config out"=w529:T1)  [unwired: 8 in]
        n357 = Concatenate Strings(w522, w522, w522, w526, w522, w524, w522, w521, "\r\n") -> (w527:string)
        n358 = Unbundle By Name(w529) -> ("File Refnum"=w528:refnum<file>)
        n359 = Bundle(w517, w518) -> (w539:cluster{dbl[], dbl[]})  [unwired: 1 in]
        n360 = Bundle(w517, w536) -> (w542:cluster{dbl[], dbl[]})  [unwired: 1 in]
        n361 = Write to Text File(file (use dialog)=w528, text=w527) -> ()  [unwired: 2 in, 3 out]
        n362 = Build Array(w542, w539) -> (→"Calibration Graph":cluster{dbl[], dbl[]}[])
      }
      frame "Close File" {
        n363 = Unbundle By Name(w561) -> ("File Refnum"=w558:refnum<file>)
        n364 = Not A Number/Path/Refnum?(number/path/refnum=w558) -> (NaN/Path/Refnum?=w557:bool)
        n365 = case shown="False" w557 {
          tunnel: w558 -> [w564 _]
          frame False {
            n366 = Close File(refnum=w564) -> ()  [unwired: 1 in, 2 out]
          }
          frame True {
          }
        }
      }
      frame "Accept" {
        w567 = "," ("string")
        w577 = path "C:/Users/Public/Documents/Calibration Data/Pumps Calibration Curves.csv" ("Pump Module Config.Settings.Pump Calibration File")
        n367 = call-poly "Enqueue Message.vi"("error in (no error)"=w590, "Message"="Close File", "Message Queue"=w591) -> ("error out"=w587:errorcluster, "dup Message Queue"=w588:refnum<queue>)  [unwired: 7 in]
        n368 = property on="Calibration Slope" class="DigNum (strict)"() -> ("Value"=w583:dbl)  [unwired: 2 in, 2 out]
        n369 = call-poly "Enqueue Message.vi"("error in (no error)"=w587, "Message"="Exit", "Message Queue"=w588) -> ("error out"=w581:errorcluster)  [unwired: 7 in, 1 out]
        n370 = call-poly <vilib>:"Read Delimited Spreadsheet.vi"("file path (dialog if empty)"=w577, "delimiter (\\t)"="\n" ("delimiter (\\t)")) -> ("all rows"=w571:string[][])  [unwired: 8 in, 5 out]
        n371 = property on="Y Intercept" class="DigNum (strict)"() -> ("Value"=w566:dbl)  [unwired: 2 in, 2 out]
        n372 = property on="File Name" class="Str"(error in=w581) -> (error out=w576:errorcluster, "Text.Text"=w574:string)  [unwired: 1 in, 1 out]
        n373 = Number To Fractional String(number=w583) -> (F-format string=w573:string)  [unwired: 3 in]
        n374 = Number To Fractional String(number=w566) -> (F-format string=w565:string)  [unwired: 3 in]
        n375 = for {
          tunnel: w574 -> [w608]
          tunnel: w571 -> [w607] mode=indexing
          tunnel: [w602] -> w570
          tunnel: [w603] -> _
          tunnel: [w601] -> w568
          i -> [w601]
          stop <- w602 stop-if-true
          n376 = Index Array(array=w607, index=0) -> (element=w604:string)
          n377 = xnode "Match Regular Expression"("input string"=w604, "regular expression"="^([^,])+") -> ("whole match"=w603:string)  [unwired: 4 in, 4 out]
          n378 = Equal?(x=w603, y=w608) -> (x = y?=w602:bool)
        }
        n379 = Concatenate Strings(w574, w567, w573, w567, w565) -> (w572:string)
        n380 = Open/Create/Replace File(file path (use dialog)=w577, error in=w576, operation (0:open)=T21."replace or create") -> (error out=w575:errorcluster)  [unwired: 3 in, 2 out]
        n381 = Build Array(w572) -> (w569:string[])
        n382 = case shown="False" w570 {
          tunnel: w571 -> [w724 w729]
          tunnel: w568 -> [_ w728]
          tunnel: [w723 w727] -> w579
          tunnel: w569 -> [w725 w726]
          frame False {
            n383 = Build Array (concatenate)(w724, w725) -> (w723:string[][])
          }
          frame True {
            n384 = Replace Array Subset(array=w729, new element=w726, index (row)=w728) -> (w727:string[][])  [unwired: 1 in]
          }
        }
        n385 = call-poly <vilib>:"Write Delimited Spreadsheet.vi"("file path (dialog if empty)"=w577, "2D data"=w579, "append to file? (new file:F)"=TRUE, "error in (no error)"=w575, "delimiter (\\t)"="," ("delimiter (\\t)")) -> ("error out"=w582:errorcluster)  [unwired: 9 in, 1 out]
      }
      frame "Decline" {
        n386 = call-poly "Enqueue Message.vi"("error in (no error)"=w734, "Message"="Close File", "Message Queue"=w736) -> ("error out"=w731:errorcluster, "dup Message Queue"=w732:refnum<queue>)  [unwired: 7 in]
        n387 = call-poly "Enqueue Message.vi"("error in (no error)"=w731, "Message"="Exit", "Message Queue"=w732) -> ("error out"=w730:errorcluster)  [unwired: 7 in, 1 out]
      }
      frame "Exit" {
        n388 = call "Close.vi"("error in (no error)"=w756, "Pump Calibration Config in"=w754) -> ("error out"=w755:errorcluster, "Pump Calibration Config out"=w749:T1)  [unwired: 8 in]
      }
    }
    n389 = node-c288() -> ()  [unwired: 1 in, 1 out]
  }
  "error out" <- w7
  "Pump Calibration Config out" <- w5
  n390 = node-c288(w3) -> ()  [unwired: 1 out]
